vi "CRYAnalysis.vi"(0 "Setup in":T3={"No.VI"=0, "Category"="", "StepName"="", "Seq setup flattened"="", "Comment"="", "Steps config."=[], "Jump config"=[], "Start"=0.0, "Increment"=0.0, "Name"="Pa", "Unit"="Pa", "Y data"=1, "Y prefix"="", "Y dB ref"=1.0, "Y unit"="", "Repeat State Array"=[]} {"Repeat State Array"."Start" format="%#_5g"; "Y dB ref" format="%.1f"; "Y data" items=["dB", "Lin"]; "Start" format="%#_5g"}, 5 "Data in":T8 {"Z data" items=["dB", "Lin"]; "X data" items=["dB", "Lin"]; "Y data" items=["dB", "Lin"]; "Z dB ref" format="%.1f"; "Z axis" items=["Log", "Lin"]; "X dB ref" format="%.1f"; "X axis" items=["Log", "Lin"]; "Y axis" items=["Log", "Lin"]; "Y dB ref" format="%.1f"; "Curve"."z" format="%.2f"; "Curve"."y" format="%.2f"; "Curve"."x" format="%.2f"}, 7 "Results in":T9 {"Margin" format="%.2f"}, 9 "Seq Setup in":string, 11 "Step name":string, 12 "Hardware in":string, 13 "Calibration in":string) -> (3 "Types Out":string[](array[string]), 4 "Inserted Names Out":string[](array[string]), 6 "Data out":T8 {"Z data" items=["dB", "Lin"]; "X data" items=["dB", "Lin"]; "Y data" items=["dB", "Lin"]; "Z dB ref" format="%.1f"; "Z axis" items=["Log", "Lin"]; "X dB ref" format="%.1f"; "X axis" items=["Log", "Lin"]; "Y axis" items=["Log", "Lin"]; "Y dB ref" format="%.1f"; "Curve"."z" format="%.2f"; "Curve"."y" format="%.2f"; "Curve"."x" format="%.2f"}, 8 "Results out":T1[](array[typedef]) {"Margin" format="%.2f"}, 10 "Wave out":T7[](array[typedef]) {"Y dB ref" format="%.1f"; "Y axis" items=["Log", "Lin"]; "Y data" items=["dB", "Lin"]; "X data" items=["dB", "Lin"]})   [LabVIEW 2013]
doc: "This VI calculates the Vrms response of a device under test to a series of stepped inputs. It is designed to be used with the create stepped sign waveform.vi. The output is a 2-D array of Vrms data. Rows refer to the channel sampled. Columns refer to each step in the test signal. The user can elect to discard some number of cycles at the beginning of each frequency."
uses:
  Typedef Control/CRYData Cluster Array.ctl
  Typedef Control/CRYData Cluster.ctl
  Typedef Control/CRYResult Cluster Array.ctl
  Typedef Control/CRYResult Cluster.ctl
  Typedef Control/CRYWaveform Cluster.ctl
  Typedef Control/CRYUnit Info Cluster.ctl
  Typedef Control/CRYCalibration 2DCluster.ctl
  Typedef Control/CRYCalibration Cluster.ctl
  Typedef Control/CRYStep.ctl
  Typedef Control/CRYStimulus Test Infor Cluster.ctl
  CRYMainGlobal.vi
  Task Sequence/CRYProject Run Control Global.vi
  Calibration/SubVI/CRYCal Global.vi
  Hardware/SubVI/CRY6175APT_Win32.dll
panel:
  out "XY Graph":cluster{dbl[], dbl[]}(graph)
  in  "Result":T1={"Name"="Test for Signal [L]", "Margin"=nan, "unit"="", "Verdict"=FALSE, "Limit"="", "Max/Min"="", "protected"=FALSE, "Step No."=0, "Test Info"="", "AutoProtect"=FALSE} {"Margin" format="%.2f"}
  in  "Datum":T2={"Name"="", "Curve"=[], "X data"=1, "Y data"=1, "Z data"=1, "X axis"=0, "Y axis"=1, "Z axis"=1, "X unit"="", "Y unit"="", "Z unit"="", "X dB ref"=1.0, "Y dB ref"=1.0, "Z dB ref"=1.0, "single val"=FALSE, "protected"=FALSE, "display X"=TRUE, "display Y"=FALSE, "display Z"=TRUE, "Test Info"="", "Step No."=0, "Plot Settings"={"Color"=0, "Interpolation"=0, "Point Style"=0, "Line Style"=0, "Point Color"=0, "Line Width"=0, "Bar Plot Style"=0, "Fill To"=0}, "AutoProtect"=FALSE} {"Z data" items=["dB", "Lin"]; "X data" items=["dB", "Lin"]; "Y data" items=["dB", "Lin"]; "Z dB ref" format="%.1f"; "Z axis" items=["Log", "Lin"]; "X dB ref" format="%.1f"; "X axis" items=["Log", "Lin"]; "Y axis" items=["Log", "Lin"]; "Y dB ref" format="%.1f"; "Curve"."z" format="%.2f"; "Curve"."y" format="%.2f"; "Curve"."x" format="%.2f"}
  out "Response Waveform":waveform(dbl)(graph)
  in  "Calibration All Cluster":T4={"Calibration"={"Calibration Step Name"="", "Device"="", "Correction Curve Name"="", "Equalization Curve Name"="", "Sensitivity Curve Name"="", "Corr Folder and File"="", "EQ Folder and File"="", "Sens Folder and File"="", "Corr Step size"=0, "EQ Step size"=0, "Input"=FALSE, "Last Cal Date (sec)"=timestamp(0 s since 1904-01-01), "Cha Name"="", "Corr Curve Found"=FALSE, "EQ Curve Found"=FALSE, "Sens Curve Found"=FALSE, "Signal Type"="", "Calibrated Device"="", "Hz"=0}, "Corr Curve"={"Name"="", "Curve"=[], "X data"=1, "Y data"=1, "Z data"=1, "X axis"=0, "Y axis"=1, "Z axis"=1, "X unit"="", "Y unit"="", "Z unit"="deg.", "X dB ref"=1.0, "Y dB ref"=1.0, "Z dB ref"=1.0, "single val"=FALSE, "protected"=FALSE, "display X"=FALSE, "display Y"=TRUE, "display Z"=TRUE, "Test Info"="", "Step No."=0, "Plot Settings"={"Color"=0, "Interpolation"=0, "Point Style"=0, "Line Style"=0, "Point Color"=0, "Line Width"=0, "Bar Plot Style"=0, "Fill To"=0}, "AutoProtect"=FALSE}, "EQ Curve"={"Name"="", "Curve"=[], "X data"=1, "Y data"=1, "Z data"=1, "X axis"=0, "Y axis"=1, "Z axis"=1, "X unit"="Hz", "Y unit"="", "Z unit"="deg.", "X dB ref"=1.0, "Y dB ref"=1.0, "Z dB ref"=1.0, "single val"=FALSE, "protected"=FALSE, "display X"=TRUE, "display Y"=TRUE, "display Z"=TRUE, "Test Info"="", "Step No."=0, "Plot Settings"={"Color"=0, "Interpolation"=0, "Point Style"=0, "Line Style"=0, "Point Color"=0, "Line Width"=0, "Bar Plot Style"=0, "Fill To"=0}, "AutoProtect"=FALSE}, "Sens Curve"={"Name"="", "Curve"=[], "X data"=1, "Y data"=1, "Z data"=1, "X axis"=0, "Y axis"=1, "Z axis"=1, "X unit"="Hz", "Y unit"="", "Z unit"="deg.", "X dB ref"=1.0, "Y dB ref"=1.0, "Z dB ref"=1.0, "single val"=FALSE, "protected"=FALSE, "display X"=TRUE, "display Y"=TRUE, "display Z"=TRUE, "Test Info"="", "Step No."=0, "Plot Settings"={"Color"=0, "Interpolation"=0, "Point Style"=0, "Line Style"=0, "Point Color"=0, "Line Width"=0, "Bar Plot Style"=0, "Fill To"=0}, "AutoProtect"=FALSE}} {"Sens Curve"."Z data" items=["dB", "Lin"]; "Sens Curve"."X data" items=["dB", "Lin"]; "Sens Curve"."Y data" items=["dB", "Lin"]; "Sens Curve"."Z dB ref" format="%.1f"; "Sens Curve"."Z axis" items=["Log", "Lin"]; "Sens Curve"."X dB ref" format="%.1f"; "Sens Curve"."X axis" items=["Log", "Lin"]; "Sens Curve"."Y axis" items=["Log", "Lin"]; "Sens Curve"."Y dB ref" format="%.1f"; "Sens Curve"."Curve"."z" format="%.2f"; "Sens Curve"."Curve"."y" format="%.2f"; "Sens Curve"."Curve"."x" format="%.2f"; "EQ Curve"."Z data" items=["dB", "Lin"]; "EQ Curve"."X data" items=["dB", "Lin"]; "EQ Curve"."Y data" items=["dB", "Lin"]; "EQ Curve"."Z dB ref" format="%.1f"; "EQ Curve"."Z axis" items=["Log", "Lin"]; "EQ Curve"."X dB ref" format="%.1f"; "EQ Curve"."X axis" items=["Log", "Lin"]; "EQ Curve"."Y axis" items=["Log", "Lin"]; "EQ Curve"."Y dB ref" format="%.1f"; "EQ Curve"."Curve"."z" format="%.2f"; "EQ Curve"."Curve"."y" format="%.2f"; "EQ Curve"."Curve"."x" format="%.2f"; "Corr Curve"."Z data" items=["dB", "Lin"]; "Corr Curve"."X data" items=["dB", "Lin"]; "Corr Curve"."Y data" items=["dB", "Lin"]; "Corr Curve"."Z dB ref" format="%.1f"; "Corr Curve"."Z axis" items=["Log", "Lin"]; "Corr Curve"."X dB ref" format="%.1f"; "Corr Curve"."X axis" items=["Log", "Lin"]; "Corr Curve"."Y axis" items=["Log", "Lin"]; "Corr Curve"."Y dB ref" format="%.1f"; "Corr Curve"."Curve"."z" format="%.2f"; "Corr Curve"."Curve"."y" format="%.2f"; "Corr Curve"."Curve"."x" format="%.2f"; "Calibration"."EQ Step size" items=["R10", "R20", "R40", "R80", "User"]; "Calibration"."Corr Step size" items=["R10", "R20", "R40", "R80", "User"]}
  out "Impulse Resp Y":dbl[][](array[numeric]) format="%.2f"
  out "Impulse Resp X":dbl[](array[numeric]) format="%.2f"
  out "Unit Info":T6
  out "Y dB ref Curve":dbl
  out "Y dB ref In":dbl
  out "Y dB ref Out":dbl
  out "Y unit Out":string
  out "Y unit In":string
  out "Sens Out":dbl format="%.2f"
  out "Freq Option":bool[](array[boolean])
  out "Channel Label In":string
  out "TSR window":u16
  in  "AC/DC":i32(slide)
  out "Stimulus Waveform":waveform(dbl)(graph)
  out "HT Option":bool[](array[boolean])
  out "Window":u16
  out "Spectrum X-axis":dbl[](array[numeric]) format="%.2f"
  in  "Manual?":bool
  in  "Y data Curve":u16(ring)=1 items=["dB", "Lin"]
  out "Y Unit Curve":string
  in  "Ref resistor":dbl format="%.2f"
  out "Sens In":dbl format="%.2f"
  out "Analysis Settings":bool
  out "Input":bool
  in  "Frequency [Hz]":dbl[](array[numeric]) format="%.2f"
  in  "cycles":u32=12
  in  "Response Data":dbl[](array[numeric]) format="%.2e"
  # "V"
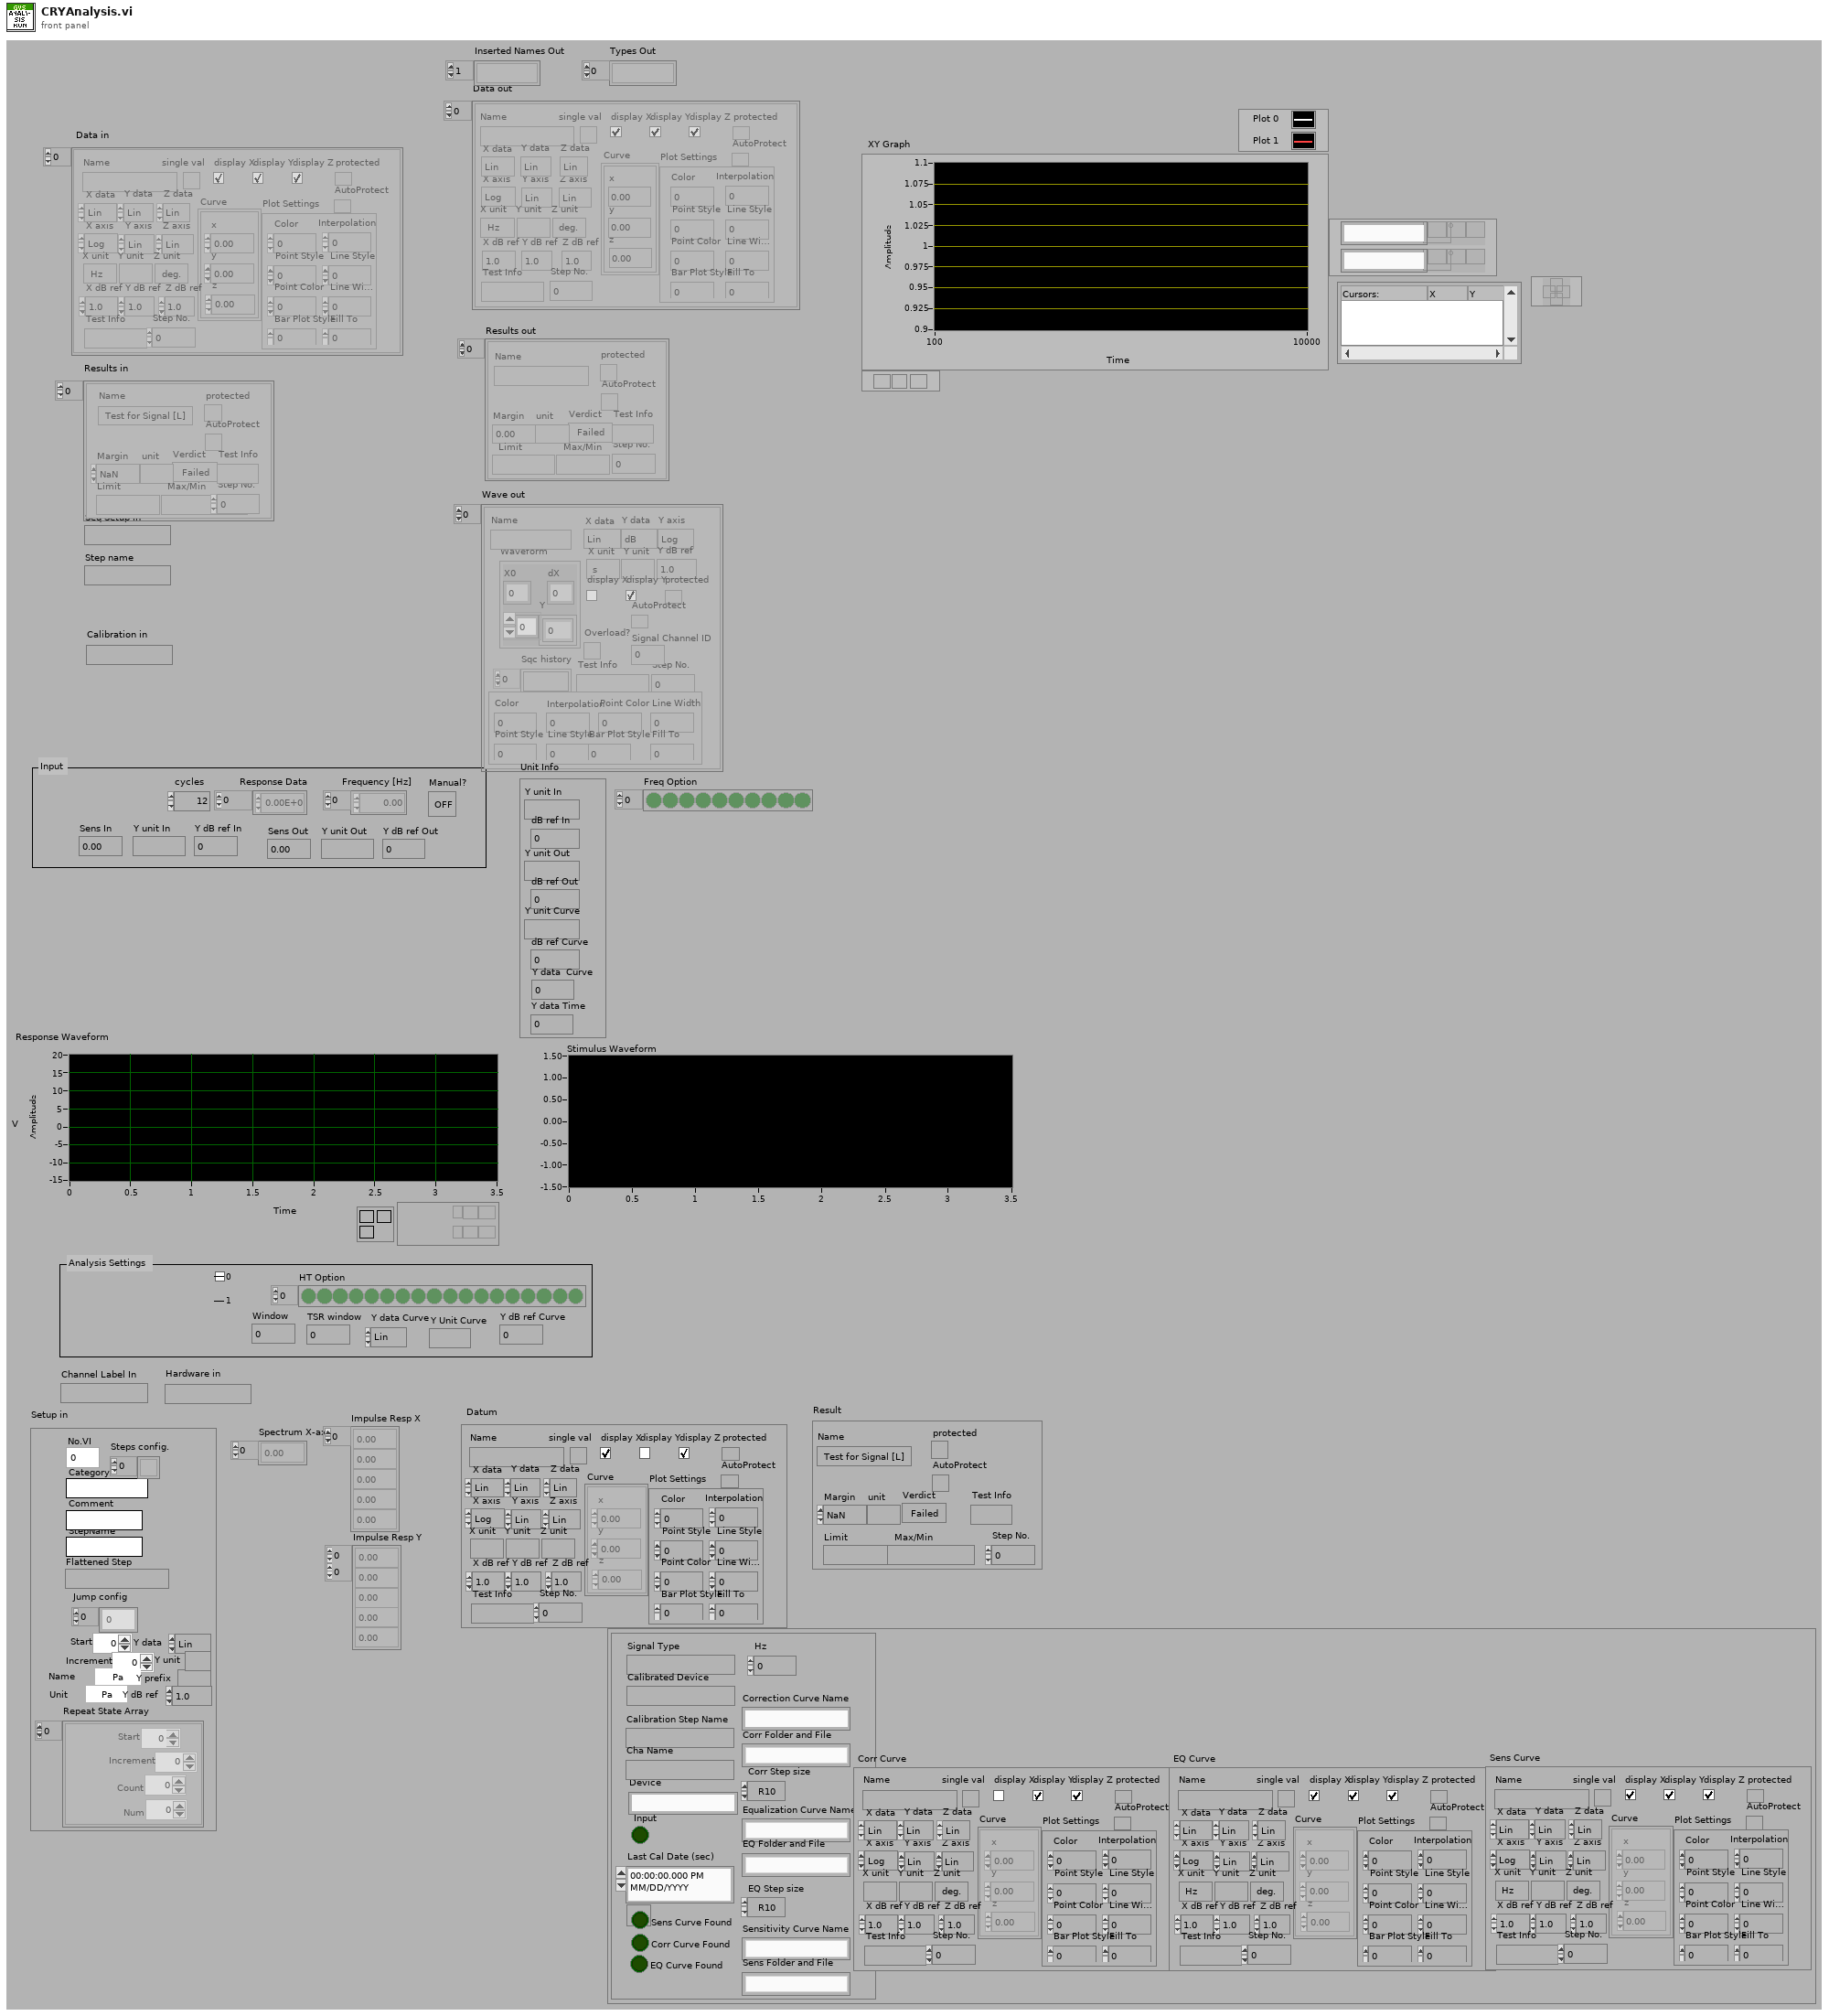
[diagram p1: front panel]
types:
  T1 = typedef "CRYResult Cluster.ctl" = cluster{"Name":string, "Margin":dbl, "unit":string, "Verdict":bool, "Limit":string, "Max/Min":string, "protected":bool, "Step No.":i32, "Test Info":string, "AutoProtect":bool}
  T2 = typedef "CRYData Cluster.ctl" = cluster{"Name":string, "Curve":cluster{"x":dbl, "y":dbl, "z":dbl}[], "X data":u16, "Y data":u16, "Z data":u16, "X axis":u16, "Y axis":u16, "Z axis":u16, "X unit":string, "Y unit":string, "Z unit":string, "X dB ref":dbl, "Y dB ref":dbl, "Z dB ref":dbl, "single val":bool, "protected":bool, "display X":bool, "display Y":bool, "display Z":bool, "Test Info":string, "Step No.":i32, "Plot Settings":cluster{"Color":u32, "Interpolation":u8, "Point Style":u8, "Line Style":u8, "Point Color":u32, "Line Width":u8, "Bar Plot Style":u8, "Fill To":i16}, "AutoProtect":bool}
  T3 = typedef "CRYStep.ctl" = cluster{"No.VI":i32, "Category":string, "StepName":string, "Seq setup flattened":string, "Comment":string, "Steps config.":bool[], "Jump config":i32[], "Start":dbl, "Increment":dbl, "Name":string, "Unit":string, "Y data":u16, "Y prefix":string, "Y dB ref":dbl, "Y unit":string, "Repeat State Array":cluster{"Start":dbl, "Increment":dbl, "Count":i32, "Num":i32}[]}
  T4 = typedef "CRYCalibration 2DCluster.ctl" = cluster{"Calibration":T5, "Corr Curve":T2, "EQ Curve":T2, "Sens Curve":T2}
  T5 = typedef "CRYCalibration Cluster.ctl" = cluster{"Calibration Step Name":string, "Device":string, "Correction Curve Name":string, "Equalization Curve Name":string, "Sensitivity Curve Name":string, "Corr Folder and File":string, "EQ Folder and File":string, "Sens Folder and File":string, "Corr Step size":u16, "EQ Step size":u16, "Input":bool, "Last Cal Date (sec)":timestamp, "Cha Name":string, "Corr Curve Found":bool, "EQ Curve Found":bool, "Sens Curve Found":bool, "Signal Type":string, "Calibrated Device":string, "Hz":u32}
  T6 = typedef "CRYUnit Info Cluster.ctl" = cluster{"Y unit In":string, "dB ref In":dbl, "Y unit Out":string, "dB ref Out":dbl, "Y unit Curve":string, "dB ref Curve":dbl, "Y data  Curve":u16, "Y data Time":u16}
  T7 = typedef "CRYWaveform Cluster.ctl" = cluster{"Waveform":cluster{"X0":dbl, "dX":dbl, "Y":sgl[]}, "X data":u16, "Y data":u16, "Y axis":u16, "X unit":string, "Y unit":string, "Y dB ref":dbl, "display Y":bool, "display X":bool, "Overload?":bool, "Test Info":string, "Step No.":i32, "Name":string, "protected":bool, "Sqc history":string[], "Signal Channel ID":i32, "Plot Settings":cluster{"Color":u32, "Interpolation":u8, "Point Style":u8, "Line Style":u8, "Point Color":u32, "Line Width":u8, "Bar Plot Style":u8, "Fill To":i16}, "AutoProtect":bool}
  T8 = typedef "CRYData Cluster Array.ctl" = T2[]
  T9 = typedef "CRYResult Cluster Array.ctl" = T1[]
  T10 = cluster{"Start":dbl, "Increment":dbl, "Count":i32, "Num":i32}[]
  T11 = enum16{"OK", "Yes", "YesNo", "YesNoCancel", "ReplaceAppend"}
  T12 = cluster{"Harmonic Track Data":cluster{cluster{"x":dbl, "y":dbl, "z":dbl}[]}[]}[]
  T13 = typedef "CRYAnalysis Cluster.ctl" = cluster{"Name":string, "Harmonics":dbl[], " Algorithm":u16, "delay":dbl, "THD(%)":bool, "Rub&Buzz":bool, "Imp":bool, "Imp Ref resistor":dbl, "Y data":u16, "Y prefix":string, "Y unit":string, "Y dB ref":dbl, "Custom Curve Names":string[], "har list items":string[], "Envelope":bool, "use custom unit":bool, "autodelay ch":dbl, "impulse":bool, " start ms":dbl, " stop ms":dbl, "Scaling":i32, "Default Overlap ":bool, "Advanced View":bool, "Loose Particle":bool, "Use default":bool, "Auto-Correlation(Stimulus)":bool, "Auto-Correlation(Response)":bool, "Deconvolved Response":bool, "Mic Current":bool, "M List Vaiues":u16, "Type":u16, "Delay Method":u16, "Apply Correction Out":bool, "Apply Correction In":bool, "Harmonics @ meas.frq":bool, "THD Normalized(%)":bool, "Total Distortion":bool, "THD+Noise(%)":bool, "Rub&Buzz Norm'd(%)":bool, "Standard Error":bool, "Confidence Limits":bool, "Total Diff":bool, "Total Noise":bool, "Total DFD(%)":bool, "Total IMD(%)":bool, "Total IM":bool, "Total DFD+Noise(%)":bool, "Use Channel Name":bool, "Waveform In":string, "Waveform Out":string, "Method":u16, "Spectral Scaling":u16, "Appliied Unit":u16, "Length Unit":u16, "Applied Units":u16, "Sens Item":u16, "Tab":i32, "Distance Unit":u16, "discard cycles":dbl, "Weigting":string, "Averaging Time":dbl, "Max duration":dbl, "Min duration":dbl, "Attack Threshold":dbl, "Hysteresis Up":dbl, "Fmin(Hz)":dbl, "Fmax(Hz)":dbl, "Freq.Resolution":dbl, "Over-samples Res.":dbl, "Win Resolution":dbl, "distance":dbl, "samples":dbl, "Overlap":dbl, "Record Length":dbl, "No.of FFTs":dbl, "Hz":dbl, "record delay":dbl, " Std Err":dbl, "Response":bool, "Coherent Power*":bool, "Stimulus":bool, "Measurement Confidence":bool, "Auto Spectrum(Response)*":bool, "Auto Spectrum(Stimulus)*":bool, "Cross Spectrum*":bool, "functions":bool, "Frequency Response":bool, "Non-Coherent Power*":bool, "Coherence (%)":bool, "Non-Coherence (%)":bool, "Signal-Noise Ratio (dB)":bool, "Non-Coherenct Distirtion*":bool, "Result Waveforms":bool, "Coupling":bool, "Averaging":u16, "Harmonics":i32, "Custom Curve Names":i32, "unLabel":string, "Custom Curve Names":string, "Unit":string, "Total IMD + Noise(%) ":bool, "ResponseMe":u16, "Intermod":dbl[], "Diff\n":dbl[], "Cross-Correlation":bool, "IM list items":string[], "Diff list items":string[], "TSR Window Type":string, "Help":string, "Custom Curve IDs":i32[], "Default Curve Names":string[], "Loose Particle waveform":bool, "Perceptual Rub&Buzz":bool, "Imp Auto Mode":u16, "Mic Auto Mode":u16, "Mic Ref resistor":dbl, "Curve Resolution":u16, "Curve Resolution Hz":dbl, "Polarity":bool}
  T14 = typedef "CRYStimulus Test Infor Cluster.ctl" = cluster{"Stimulus Type":string, "Signal Type":string, "In/Out":bool, "FAPS":cluster{"freq":dbl, "ampl":dbl, "cycles":dbl, "samples":i32}[], "Sampling Rate":dbl, "Samples":i32, "Analysis Param":string, "Resolution":u16, "Steps":u32, "Analysis Value":dbl[], "Diff Freq":dbl, "FStart":dbl, "FStop":dbl, "Calibration Param":string, "Anti Alias":dbl, "Level Out1":dbl, "Level Out2":dbl, "EQ":bool}
  T15 = cluster{bool, "Check Option":string, "use custom unit":bool, "Custom Curve Names":string[], "Custom Curve IDs":i32[], "Default Curve Names":string[], "Use default":bool}
  T16 = cluster{"freq":dbl, "ampl":dbl, "cycles":dbl, "samples":i32}[]
  T17 = cluster{"Y unit":string, "Y dB ref":dbl, "Y unit":string, "Y dB ref":dbl, "Y unit":string, "Y dB ref":dbl, "Y data":u16, u16}
  T18 = cluster{"Sampling Rate":dbl, "discard cycles":dbl, "Sens In":dbl, "AC/DC":i32}
  T19 = cluster{"Window":u16, "Freq.Resolution":dbl, "Overlap":dbl, "Spectral Scaling":u16, "Sens In":dbl}
  T20 = cluster{"EQ Curve":T2, "EQ":bool, "Level Out2":dbl}
  T21 = cluster{"ResponseMe":u16, "Sampling Rate":dbl, "Sens In":dbl}
  T22 = cluster{dbl[], "Frequency [Hz]":dbl[], dbl[], bool, "Diff Freq":dbl}
  T23 = cluster{"Type":u16, "Method":u16, "HT Option":bool[], "Harmonics array out":dbl[], bool, "Apply Correction In":bool, " Std Err":dbl}
  T24 = cluster{dbl[], "Frequency [Hz]":dbl[], dbl[], i32[], "Sampling Rate":dbl, "Window":u16, "discard cycles":dbl}
  T25 = cluster{"FSamp":dbl, "FStart":dbl, "FStop":dbl, "NOffset":dbl, "MStop":dbl, "MStart":dbl, "NHarm":dbl, "Tsamp":dbl, "Amplit":dbl, "Amplit 2":dbl}
  T26 = cluster{"TSR Window Type":string, " start ms":dbl, " stop ms":dbl, "Over-samples Res.":dbl}
  T27 = cluster{dbl[], dbl[], dbl[], i32[], "Sampling Rate":dbl, "Window":u16, "Sampling Rate":dbl}
  T28 = cluster{"Curve Resolution Hz":dbl, "Overlap":dbl, "Window":u16}
  T29 = cluster{"display X":bool, "display Y":bool, "display Z":bool}[]
  T30 = typedef "CRYUnit Info Out Cluster.ctl" = cluster{"X unit":string, "X data":u16, "Y unit":string, "Y data Time":u16, "Z unit":string, "X axis":u16, "X dB ref":dbl, "Y dB ref":dbl, "single/curve":bool}
  T31 = typedef "CRYAnalysis CurveName Cluster.ctl" = cluster{"Custom Curve Name":string, "Custom Curve ID":i32, "Default Curve Name":string}[]
  T32 = cluster{bool, "Check Option":string, bool, "Custom Curve Names":string[], "Custom Curve IDs":i32[], "Default Curve Names":string[], "Use default":bool}
  T33 = cluster{"display X":bool, "display Y":bool, "display Z":bool}
  T34 = cluster{"Harmonics array out":dbl[], "Impulse Resp X":dbl[], "Impulse Resp Y":dbl[][]}
  T35 = cluster{"Fmin(Hz)":dbl, "Fmax(Hz)":dbl, "Averaging":u16, "Scaling":i32}
  T36 = cluster{"Sampling Rate":dbl, "Channel Label In":string, "Make Fundamental curve?":bool}
  T37 = cluster{"Window":u16, "TSR window":u16, "Freq.Resolution":dbl, "Default Overlap ":bool, "Overlap":dbl, "discard cycles":dbl, " start ms":dbl, " stop ms":dbl, "Over-samples Res.":dbl, "ResponseMe":u16, "Weigting":string}
  T38 = cluster{bool, string, "use custom unit":bool, "Custom Curve Names":string[], "Custom Curve IDs":i32[], "Default Curve Names":string[], "Use default":bool}
  T39 = cluster{"Attack Threshold":dbl, "Averaging Time":dbl, "Max duration":dbl, "Min duration":dbl, "Hysteresis Up":dbl, "Loose Particle":bool}
  T40 = typedef "CRYWaveform Cluster Array.ctl" = T7[]
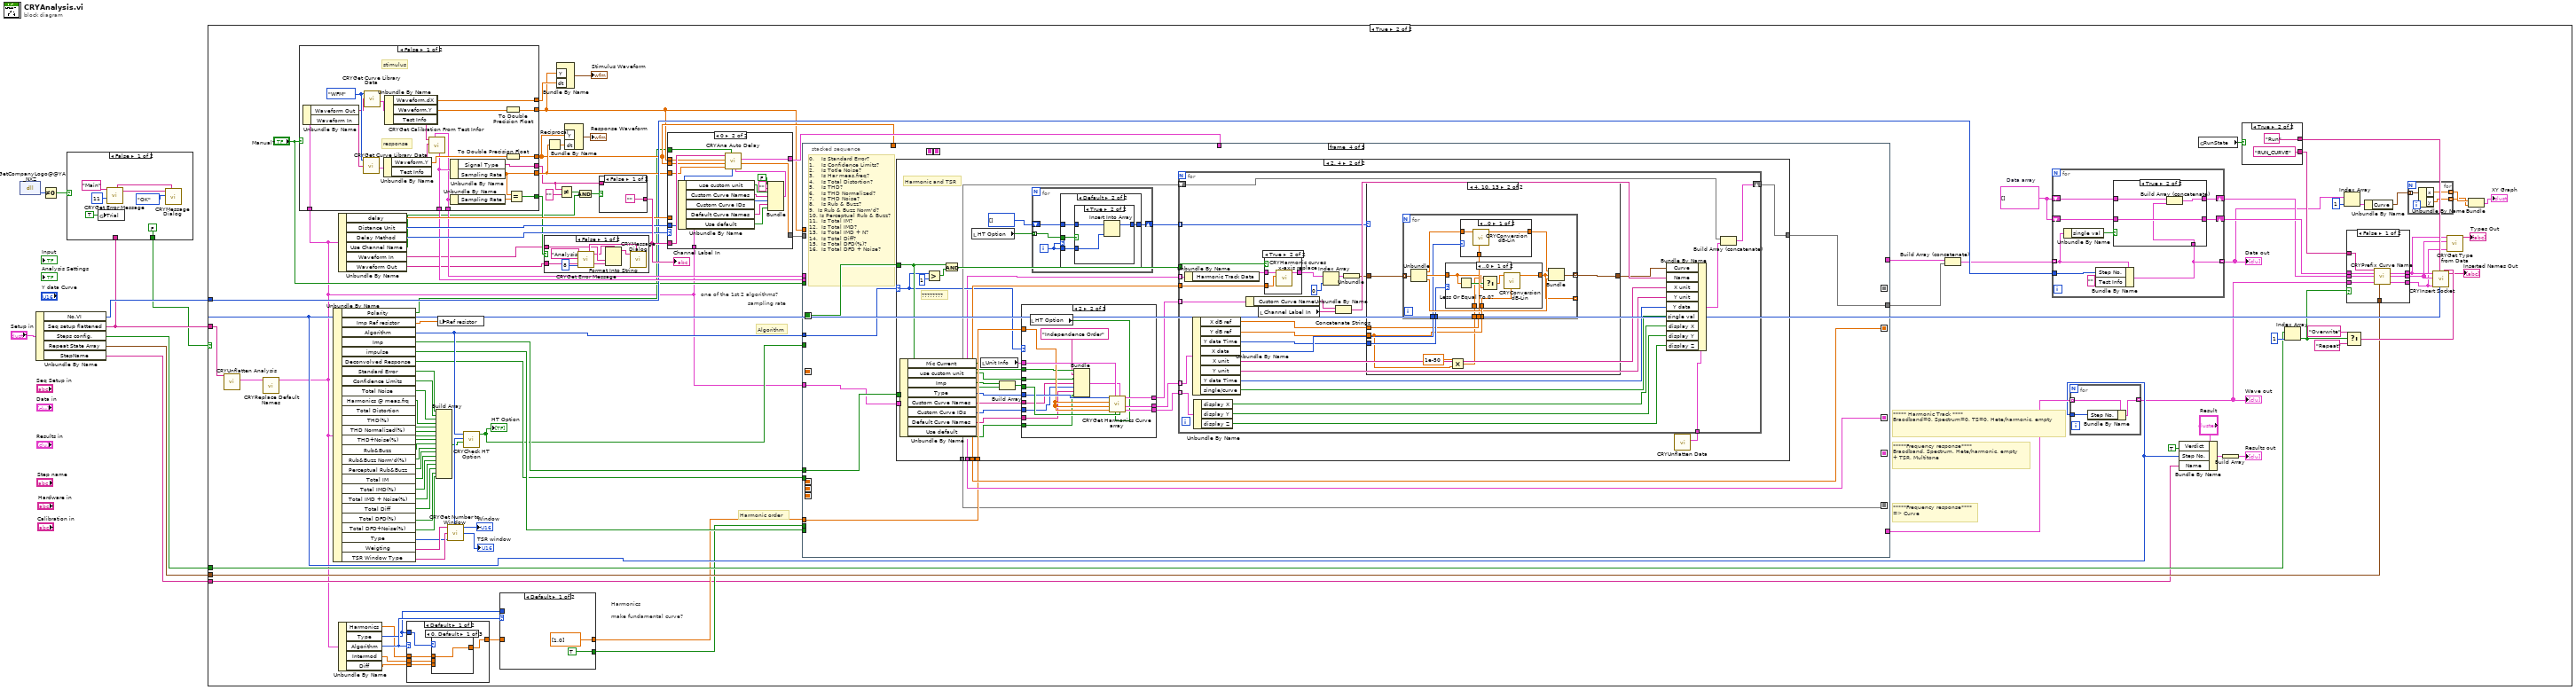
[diagram p0: block diagram]
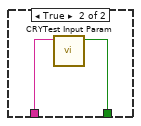
[diagram p2: hidden frame]
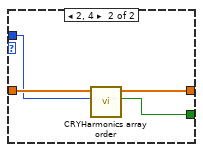
[diagram p4: hidden frame]
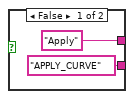
[diagram p6: hidden frame]
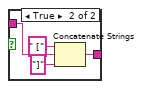
[diagram p8: hidden frame]
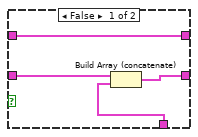
[diagram p9: hidden frame]
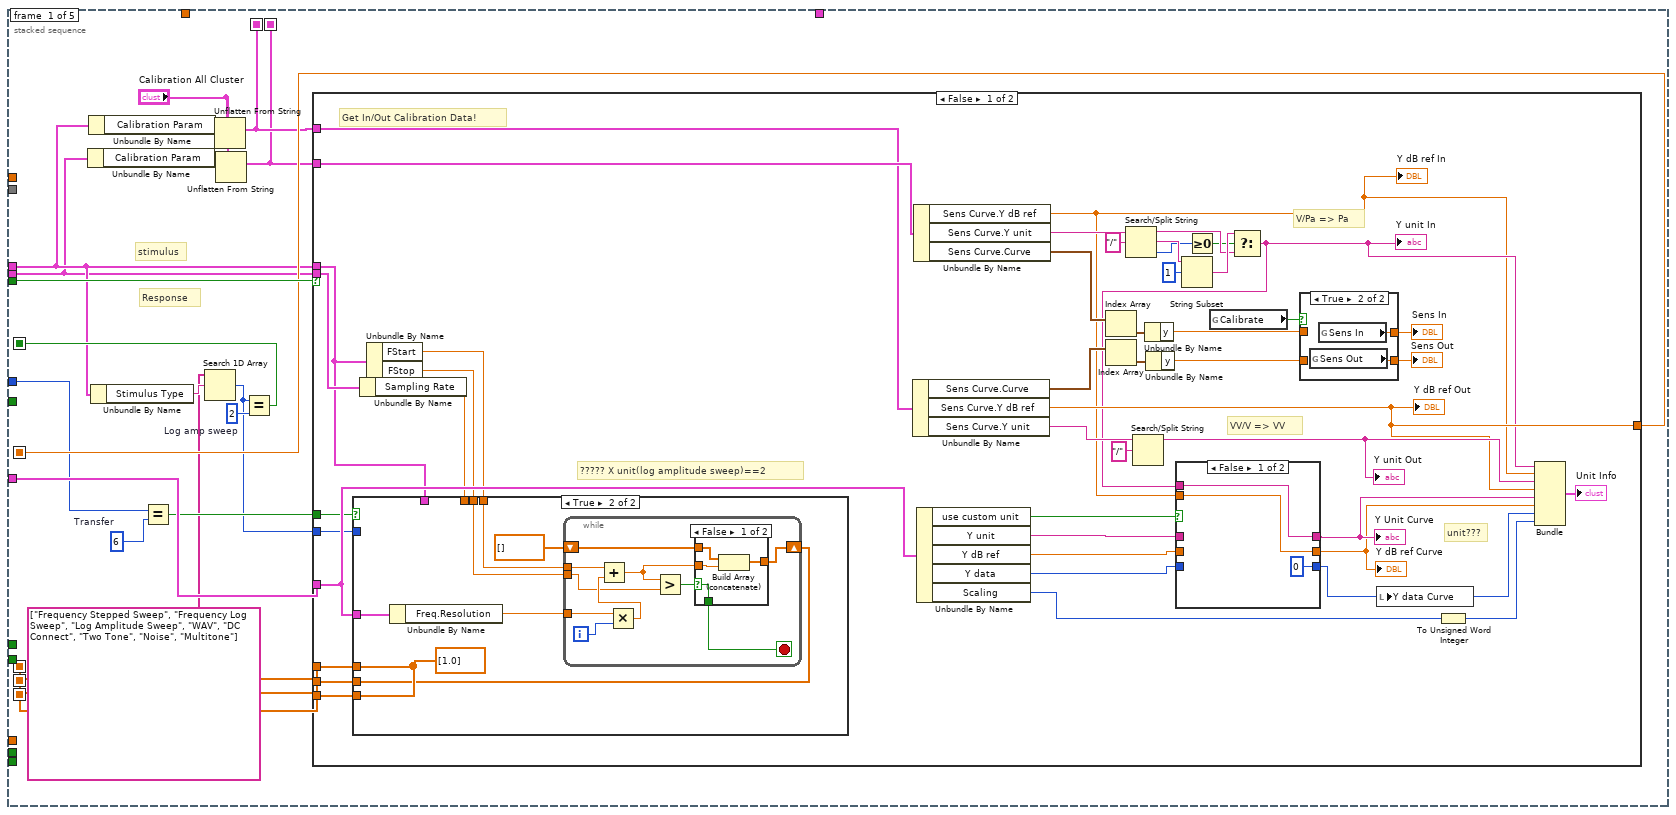
[diagram p10: hidden frame]
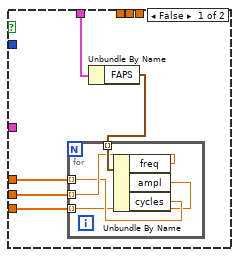
[diagram p11: hidden frame]
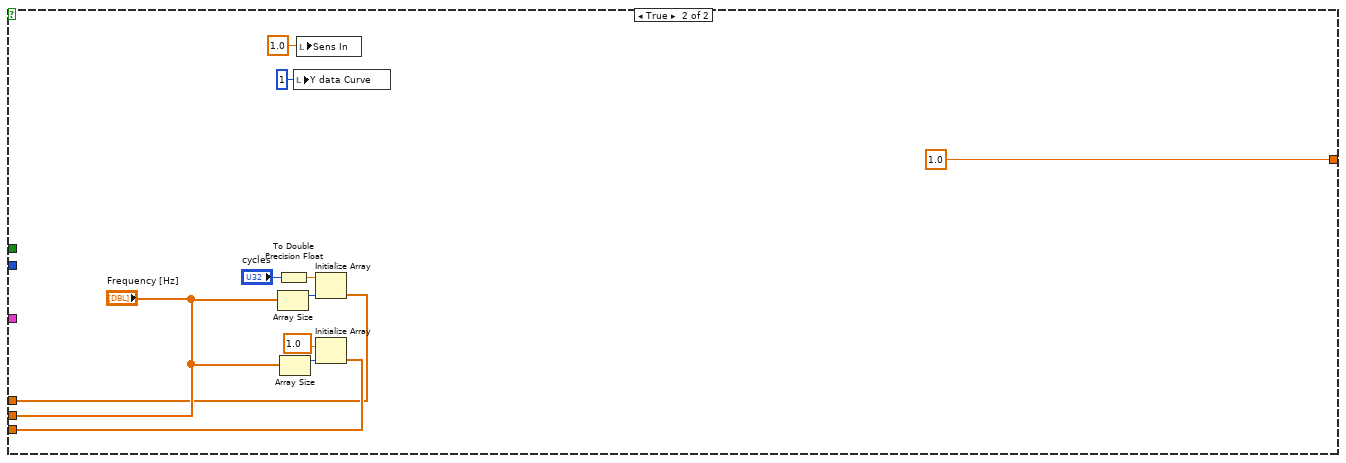
[diagram p15: hidden frame]
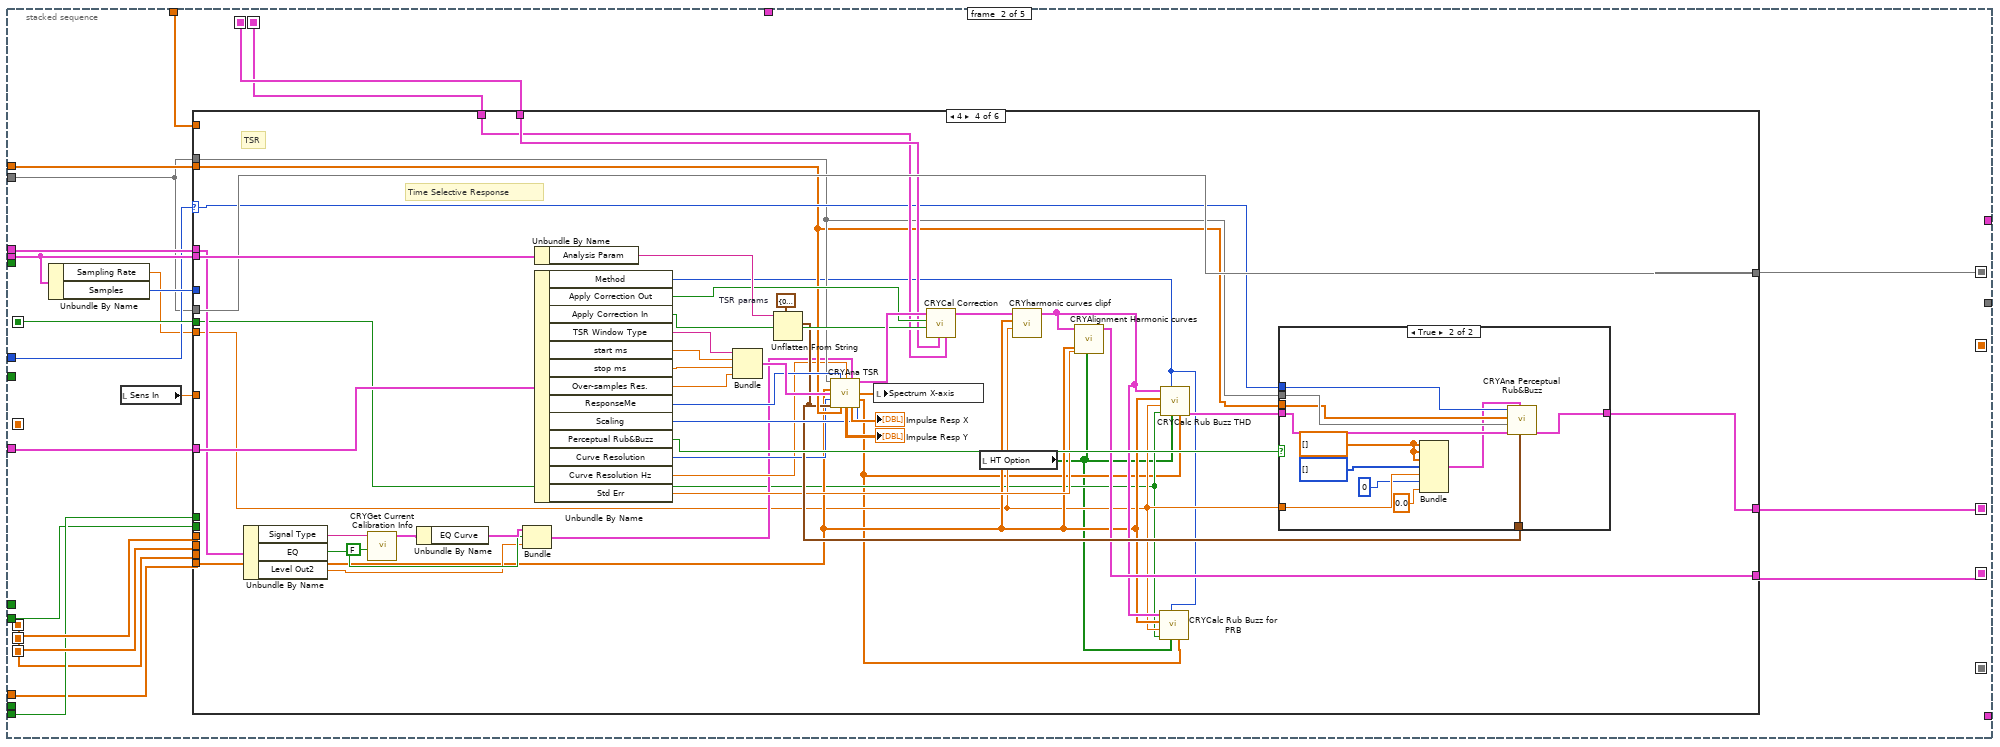
[diagram p16: hidden frame]
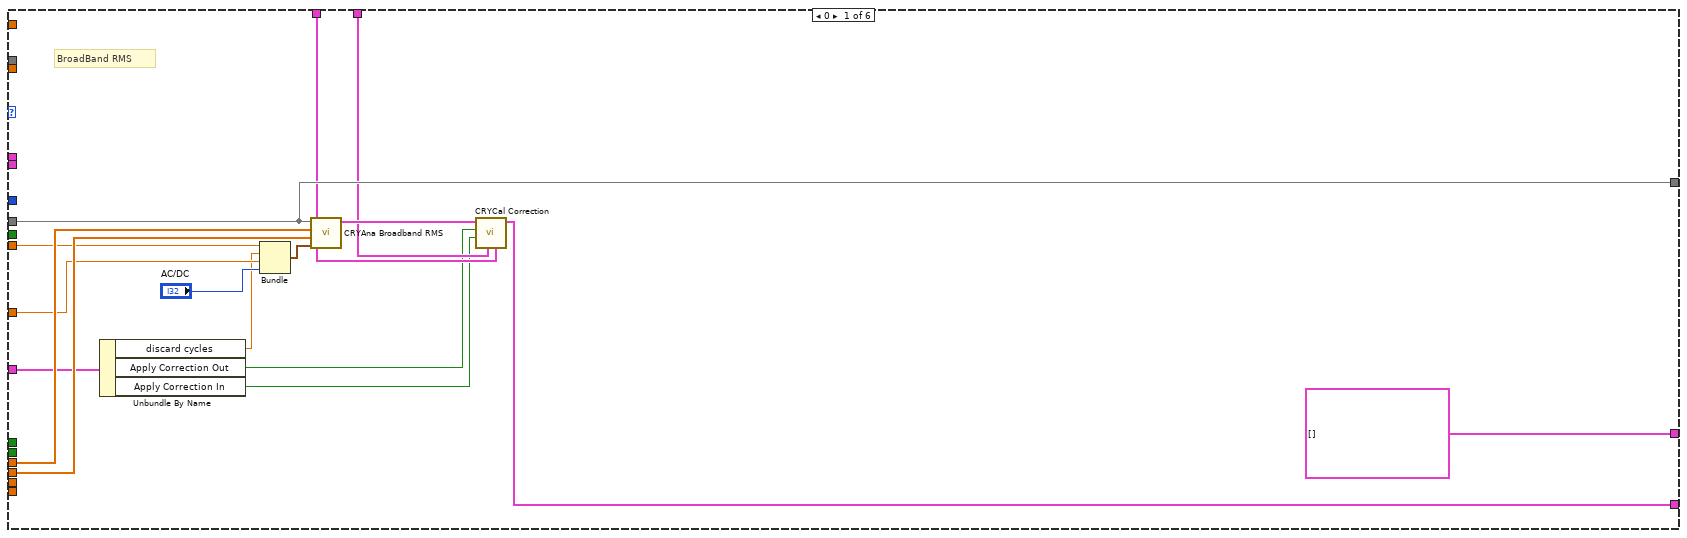
[diagram p17: hidden frame]
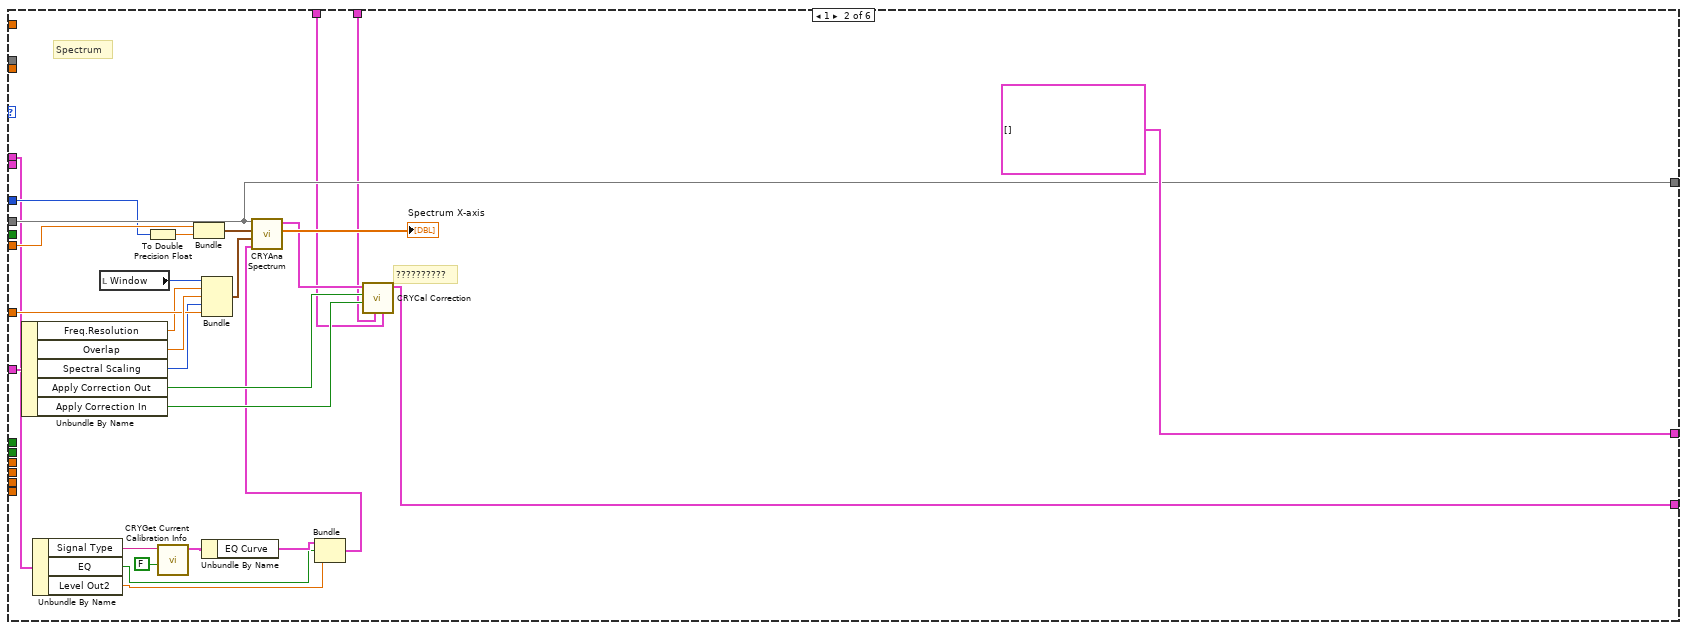
[diagram p18: hidden frame]
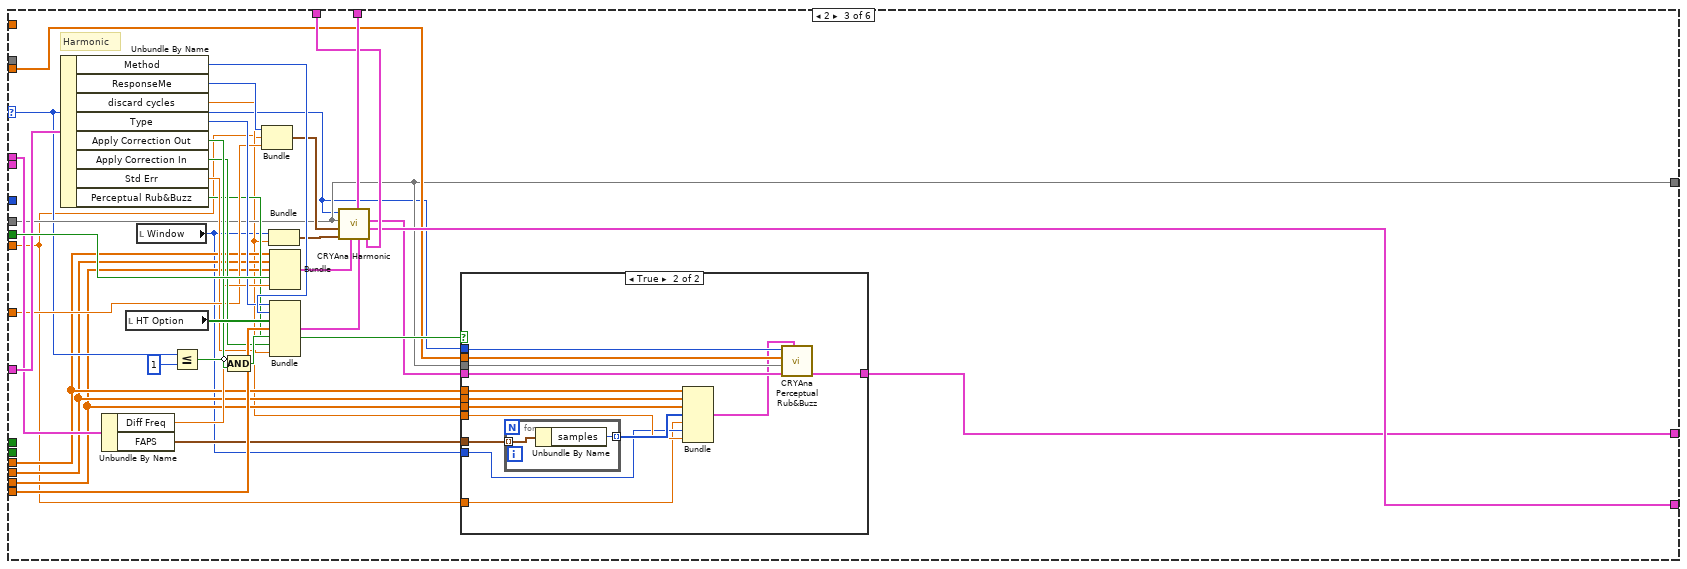
[diagram p19: hidden frame]
diagram:
  n1 = dll-call lib="D:/A_CRYSoundLab_Work/CRY6181/CRYSystem/Hardware/SubVI/CRY6175APT_Win32.dll" fn="?GetCompanyLogo@@YA_NXZ"() -> ("return type"=w4:i32)  [unwired: 3 in, 2 out]
  n2 = Unbundle By Name("Setup in") -> ("No.VI"=w9:i32, "Seq setup flattened"=w2:string, "Steps config."=w8:bool[], "Repeat State Array"=w7:T10, "StepName"=w6:string)
  n3 = Not Equal To 0?(x=w4) -> (x != 0?=w3:bool)
  n4 = case shown="False" w3 {
    tunnel: w2 -> [_ w18]
    tunnel: [FALSE ("test result") w17] -> w1
    frame False {
      n5 = global write "CRYMainGlobal.vi" "Trial"(TRUE ("Trial")) -> ()
      n6 = call "CRYGet Error Message.vi"("Error No"=11, "Kind"="Main") -> ("Message"=w11:string, "Window Title"=w15:string)  [unwired: 4 in, 4 out]
      n7 = call "CRYMessage Dialog.vi"("Window Title"=w15, "YesNoCancel"=T11."OK", "Message Content"=w11) -> ()  [unwired: 7 in, 2 out]
    }
    frame True {
      n8 = call "CRYTest Input Param.vi"("Flattend Analysis"=w18) -> ("test result"=w17:bool)  [unwired: 10 out]
    }
  }
  n9 = case shown="True" w1 {
    tunnel: w9 -> [_ w101]
    tunnel: w8 -> [_ w97]
    tunnel: w7 -> [_ w90]
    tunnel: w6 -> [_ w45]
    tunnel: w2 -> [_ w27]
    frame False {
    }
    frame True {
      w48 = T8 []  # Data array
      # "make fundamental curve?"
      # "Harmonics"
      # "*****Frequency response****\n=> Curve"
      # "***** Harmonic Track ****\nBraodband=0, Spectrum=0, TS=0, Hete/harmonic, empty"
      # "*****Frequency response****\nBraodband, Spectrum, Hete/harmonic, empty\n+ TSR, Multitone"
      # "Harmonic order"
      # "sampling rate"
      # "Algorithm"
      # "one of the 1st 2 algorithms?"
      n10 = call "CRYUnflatten Analysis.vi"("Unflatten Analysis"=w27) -> ("Analysis"=w25:T13)  [unwired: 10 out]
      n11 = call "CRYReplace Default Names.vi"("Analysis In"=w25) -> ("Analysis Out"=w24:T13)  [unwired: 10 in]
      n12 = case shown="False" "Manual?" {
        tunnel: [w1181 "Response Data"] -> w29
        tunnel: [w1182 "Response Data"] -> w94
        tunnel: w24 -> [w1180 _]
        tunnel: [w1179 "" ("Stimulus Type")] -> w22
        tunnel: [w1174 44100.0 ("Sampling Rate")] -> w95
        tunnel: [w1177 w1192] -> w103
        tunnel: [w1175 w1192] -> w102
        tunnel: [w1172 TRUE] -> w86
        tunnel: [w1171 44100.0 ("Sampling Rate")] -> w30
        frame False {
          w1187 = enum16{"Curves", "Values", "Results", "WFM"}."WFM" ("Type")
          # "response"
          # "stimulus"
          n13 = Unbundle By Name(w1180) -> ("Waveform Out"=w1185:string, "Waveform In"=w1186:string)
          n14 = call "CRYGet Curve Library Data.vi"("Type"=w1187, "Data Name"=w1186) -> ("Wave"=w1189:T7)  [unwired: 4 out]
          n15 = call "CRYGet Curve Library Data.vi"("Type"=w1187, "Data Name"=w1185) -> ("Wave"=w1188:T7)  [unwired: 4 out]
          n16 = Unbundle By Name(w1189) -> ("Waveform.Y"=w1183:sgl[], "Test Info"=w1176:string)
          n17 = Unbundle By Name(w1188) -> ("Waveform.dX"=w1171:dbl, "Waveform.Y"=w1184:sgl[], "Test Info"=w1178:string)
          n18 = call "CRYGet Calibration From Test Infor.vi"("Response Test Information Flatten"=w1176, "Stimulus Test Information Flatten"=w1178) -> ("unflattened Response test infor data"=w1177:T14, "unflattened Stimulus test infor data"=w1175:T14)  [unwired: 5 in, 3 out]
          n19 = Unbundle By Name(w1177) -> ("Signal Type"=w1179:string, "Sampling Rate"=w1174:dbl)
          n20 = Unbundle By Name(w1175) -> ("Sampling Rate"=w1173:dbl)
          n21 = To Double Precision Float(number=w1184) -> (double precision float=w1181:dbl[])
          n22 = To Double Precision Float(number=w1183) -> (double precision float=w1182:dbl[])
          n23 = Equal?(x=w1174, y=w1173) -> (x = y?=w1172:bool)
        }
        frame True {
          w1192 = T14 {"Stimulus Type"="", "Signal Type"="", "In/Out"=FALSE, "FAPS"=[], "Sampling Rate"=0.0, "Samples"=0, "Analysis Param"="", "Resolution"=0, "Steps"=0, "Analysis Value"=[], "Diff Freq"=0.0, "FStart"=0.0, "FStop"=0.0, "Calibration Param"="", "Anti Alias"=0.0, "Level Out1"=0.0, "Level Out2"=0.0, "EQ"=FALSE}  # unflattened test infor cluster
        }
      }
      n24 = Unbundle By Name(w24) -> ("Polarity"=w26:bool, "Imp Ref resistor"=w74:dbl, "Algorithm"=w119:u16, "Imp"=w107:bool, "impulse"=w118:bool, "Deconvolved Response"=w113:bool, "Standard Error"=w73:bool, "Confidence Limits"=w72:bool, "Total Noise"=w71:bool, "Harmonics @ meas.frq"=w70:bool, "Total Distortion"=w69:bool, "THD(%)"=w68:bool, "THD Normalized(%)"=w67:bool, "THD+Noise(%)"=w66:bool, "Rub&Buzz"=w65:bool, "Rub&Buzz Norm'd(%)"=w64:bool, "Perceptual Rub&Buzz"=w31:bool, "Total IM"=w63:bool, "Total IMD(%)"=w62:bool, "Total IMD + Noise(%)"=w61:bool, "Total Diff"=w60:bool, "Total DFD(%)"=w59:bool, "Total DFD+Noise(%)"=w58:bool, "Type"=w53:u16, "Weigting"=w55:string, "TSR Window Type"=w54:string)
      n25 = Unbundle By Name(w24) -> ("delay"=w109:dbl, "Distance Unit"=w104:u16, "Delay Method"=w108:u16, "Use Channel Name"=w19:bool, "Waveform In"=w85:string, "Waveform Out"=w84:string)
      n26 = Unbundle By Name(w24) -> ("Harmonics"=w77:dbl[], "Type"=w80:u16, "Algorithm"=w81:u16, "Intermod"=w78:dbl[], "Diff"=w82:dbl[])
      n27 = case shown="Default" w81 {
        tunnel: w77 -> [w1200 w1204]
        tunnel: w78 -> [w1199 _]
        tunnel: w82 -> [w1198 _]
        tunnel: [w1197 w1204] -> w79
        tunnel: w80 -> [w1196 _]
        frame Default {
          n28 = case shown="0, Default" w1196 {
            tunnel: w1200 -> [w1201 _ _]
            tunnel: [w1201 w1202 w1203] -> w1197
            tunnel: w1199 -> [_ w1202 _]
            tunnel: w1198 -> [_ _ w1203]
            frame 0, Default {
            }
            frame 1 {
            }
            frame 2 {
            }
          }
        }
        frame 4 {
        }
      }
      n29 = Build Array(w73, w72, w71, w70, w69, w68, w67, w66, w65, w64, w31, w63, w62, w61, w60, w59, w58) -> (w52:bool[])
      n30 = local write "Ref resistor"(w74) -> ()
      n31 = call "CRYGet Number to Window.vi"("TSR Window Name"=w54, "Weighting Name"=w55) -> ("TSR window"=→"TSR window":u16, "Weighting"=→"Window":u16)  [unwired: 2 in]
      n32 = call "CRYCheck HT Option.vi"("Option Array In"=w52, "Type"=w53, "Algorithm"=w119) -> ("Option Array Out"=w51:bool[])  [unwired: 8 in]
      "HT Option" <- w51
      n33 = case shown="Default" w81 {
        tunnel: [dbl[] [1.0] ("Harmonics") w128] -> w76
        tunnel: w79 -> [_ w126]
        tunnel: [TRUE ("Make Fundamental curve?") w127] -> w75
        tunnel: w80 -> [_ w125]
        frame Default {
        }
        frame 2, 4 {
          n34 = call "CRYHarmonics array order.vi"("Type"=w125, "Harmonics array in"=w126) -> ("Make Fundamental curve?"=w127:bool, "Harmonics array out"=w128:dbl[])  [unwired: 8 out]
        }
      }
      n35 = case shown="False" w86 {
        tunnel: w85 -> [w131 _]
        tunnel: w84 -> [w130 _]
        frame False {
          n36 = call "CRYGet Error Message.vi"("Error No"=8, "Kind"="Analysis") -> ("Message"=w129:string, "Window Title"=w133:string)  [unwired: 4 in, 4 out]
          n37 = Format Into String(format string=w129, w131, w130) -> (resulting string=w132:string)  [unwired: 2 in, 1 out]
          n38 = call "CRYMessage Dialog.vi"("Window Title"=w133, "Message Content"=w132) -> ()  [unwired: 8 in, 2 out]
        }
        frame True {
        }
      }
      n39 = Reciprocal(x=w95) -> (1/x=w46:dbl)
      n40 = Bundle By Name("Y"=w29, "dt"=w30) -> (→"Stimulus Waveform":waveform(dbl))  [unwired: 1 in]
      n41 = Not Equal?(x=w22, y="") -> (x != y?=w20:bool)
      n42 = Bundle By Name("Y"=w94, "dt"=w46) -> (→"Response Waveform":waveform(dbl))  [unwired: 1 in]
      n43 = And(x=w20, y=w19) -> (x .and. y?=w21:bool)
      n44 = case shown="False" w21 {
        tunnel: w22 -> [_ w153]
        tunnel: ["" w152] -> w112
        frame False {
        }
        frame True {
          n45 = Concatenate Strings(" [" ("string"), w153, "]" ("string")) -> (w152:string)
        }
      }
      "Channel Label In" <- w112
      n46 = case shown="0" w108 {
        tunnel: w95 -> [w1153 w1167]
        tunnel: w29 -> [_ w1169]
        tunnel: w94 -> [w1152 w1168]
        tunnel: [w1150 w1165] -> w114
        tunnel: [w1147 w1155] -> w106
        tunnel: w112 -> [_ w1170]
        tunnel: w104 -> [_ w1166]
        tunnel: w109 -> [w1149 _]
        tunnel: w24 -> [_ w1164]
        tunnel: w26 -> [_ w1154]
        frame Default {
          (unwired) 0.001
          # "Fs * t * 0.001"
          # "??????"
          n47 = Compound Arithmetic op=MULTIPLY(w1153, w1149) -> (w1151:dbl)
          n48 = Array Subset(array=w1152, index=w1151) -> (w1150:dbl[])  [unwired: 1 in]
          n49 = Initialize Array("Datum", 0 ("dimension size")) -> (w1147:T2[])
        }
        frame 0 {
          n50 = Unbundle By Name(w1164) -> ("use custom unit"=w1158:bool, "Custom Curve Names"=w1159:string[], "Custom Curve IDs"=w1160:i32[], "Default Curve Names"=w1161:string[], "Use default"=w1163:bool)
          n51 = Bundle(FALSE, "Check Option"="", "use custom unit"=w1158, "Custom Curve Names"=w1159, "Custom Curve IDs"=w1160, "Default Curve Names"=w1161, "Use default"=w1163) -> (w1162:T15)  [unwired: 1 in]
          n52 = call "CRYAna Auto Delay.vi"("Additive Info"=w1162, "Distance Unit"=w1166, "Polarity"=w1154, "Fs"=w1167, "Response"=w1168, "Stimulus"=w1169, "Channel Name"=w1170) -> ("Result Response"=w1165:dbl[], "Value Out"=w1155:T2[])  [unwired: 2 in, 1 out]
        }
      }
      n53 = stacked-sequence {
        seq-local: [w196 _ _ _ _] -> [_ w317 w591 _ _]
        seq-local: [w195 _ _ _ _] -> [_ w316 _ _ _]
        seq-local: [w194 _ _ _ _] -> [_ w311 w586 _ _]
        seq-local: [_ w297 _ _ _] -> [_ _ w577 _ _]
        seq-local: [w191 _ _ _ _] -> [_ w315 w572 w920 w1087]
        seq-local: [w192 _ _ _ _] -> [_ _ w584 _ _]
        seq-local: [_ w312 _ _ _] -> [_ _ _ w919 _]
        seq-local: [_ _ w583 _ _] -> [_ _ _ w921 _]
        seq-local: [_ _ w566 _ _] -> [_ _ _ w914 _]
        seq-local: [_ w307 _ _ _] -> [_ _ _ _ _]
        seq-local: [w180 _ _ _ _] -> [_ w304 _ _ _]
        seq-local: [w179 _ _ _ _] -> [_ w303 _ _ _]
        tunnel: [_ _ _ w915 _] -> w117
        tunnel: "Manual?" -> [w193 _ _ _ _]
        tunnel: w119 -> [w187 w301 w576 w916 w1101]
        tunnel: w114 -> [_ w299 _ _ _]
        tunnel: w118 -> [_ w314 _ _ _]
        tunnel: w76 -> [_ w296 w582 w917 w1102]
        tunnel: w75 -> [_ _ w573 _ w1100]
        tunnel: w24 -> [w189 w308 w579 w913 w1085]
        tunnel: [_ _ _ _ w1075] -> w115
        tunnel: w113 -> [_ w313 _ _ _]
        tunnel: w29 -> [_ w310 _ _ w1093]
        tunnel: w107 -> [_ _ _ w918 _]
        tunnel: w106 -> [_ _ _ _ w1097]
        tunnel: [_ _ _ _ w1076] -> w105
        tunnel: w94 -> [_ w300 _ _ w1078]
        tunnel: w103 -> [w181 w302 w559 _ w1091]
        tunnel: w102 -> [w182 w305 _ _ w1069]
        tunnel: w51 -> [_ _ _ _ _]
        frame #0 {
          w188 = u16 6  # Transfer
          w190 = 2  # Log amp sweep
          # "Response"
          # "stimulus"
          # "cycle\nfreq\namp"
          n54 = Unbundle By Name(w181) -> ("Calibration Param"=w183:string)
          n55 = Unbundle By Name(w182) -> ("Calibration Param"=w184:string)
          n56 = Unbundle By Name(w182) -> ("Stimulus Type"=w185:string)
          n57 = Equal?(x=w187, y=w188) -> (x = y?=w186:bool)
          n58 = Search 1D Array(1D array=string[] ["Frequency Stepped Sweep", "Frequency Log Sweep", "Log Amplitude Sweep", "WAV", "DC Connect", "Two Tone", "Noise", "Multitone"] ("Strings []"), element=w185) -> (index of element=w178:i32)  [unwired: 1 out]
          n59 = Unflatten From String(type="Calibration All Cluster", binary string=w184) -> (value=w180:T4)  [unwired: 2 in, 3 out]
          n60 = Unflatten From String(type="Calibration All Cluster", binary string=w183) -> (value=w179:T4)  [unwired: 2 in, 3 out]
          n61 = Equal?(x=w178, y=w190) -> (x = y?=w191:bool)
          n62 = case shown="False" w193 {
            tunnel: [w234 w287] -> w195
            tunnel: [w236 "Frequency [Hz]"] -> w196
            tunnel: [w235 w291] -> w194
            tunnel: [w216 1.0 ("dB Ref Out")] -> w192
            tunnel: w189 -> [w215 _]
            tunnel: w186 -> [w214 _]
            tunnel: w182 -> [w211 _]
            tunnel: w181 -> [w212 _]
            tunnel: w180 -> [w208 _]
            tunnel: w179 -> [w209 _]
            tunnel: w178 -> [w207 _]
            frame False {
              # "unit???"
              # "V/Pa => Pa"
              # "VV/V => VV"
              # "????? X unit(log amplitude sweep)==2"
              # "Get In/Out Calibration Data!"
              n63 = Unbundle By Name(w212) -> ("Sampling Rate"=w210:dbl)
              n64 = Unbundle By Name(w211) -> ("FStart"=w213:dbl, "FStop"=w206:dbl)
              n65 = case shown="True" w214 {
                tunnel: [w247 w252] -> w236
                tunnel: [w246 w257] -> w235
                tunnel: [w245 w257] -> w234
                tunnel: w215 -> [_ w258]
                tunnel: w210 -> [_ _]
                tunnel: w213 -> [_ w256]
                tunnel: w211 -> [w244 _]
                tunnel: w207 -> [_ _]
                tunnel: w206 -> [_ w255]
                frame False {
                  n66 = Unbundle By Name(w244) -> ("FAPS"=w243:T16)
                  n67 = for {
                    tunnel: w243 -> [w251] mode=indexing
                    tunnel: [w250] -> w247 mode=indexing
                    tunnel: [w248] -> w246 mode=indexing
                    tunnel: [w249] -> w245 mode=indexing
                    n68 = Unbundle By Name(w251) -> ("freq"=w250:dbl, "ampl"=w248:dbl, "cycles"=w249:dbl)
                  }
                }
                frame True {
                  w257 = dbl[] [1.0]
                  n69 = Unbundle By Name(w258) -> ("Freq.Resolution"=w254:dbl)
                  n70 = while {
                    tunnel: w256 -> [w266]
                    tunnel: w255 -> [w261]
                    tunnel: w254 -> [w267]
                    shift-right: [w263] -> w252
                    shift-left: dbl[] [] ("appended array") -> [w264]
                    i -> [w268]
                    stop <- w259 stop-if-true
                    n71 = Multiply(x=w267, y=w268) -> (x*y=w265:dbl)
                    n72 = Add(x=w266, y=w265) -> (x+y=w260:dbl)
                    n73 = Greater?(x=w260, y=w261) -> (0:w262:bool)
                    n74 = case shown="False" w262 {
                      selector: w262 -> [w270 w273]
                      tunnel: [w271 w274] -> w263
                      tunnel: w264 -> [w272 w274]
                      tunnel: [w270 w273] -> w259
                      tunnel: w260 -> [w269 _]
                      frame False {
                        n75 = Build Array (concatenate)(w272, w269) -> (w271:dbl[])
                      }
                      frame True {
                      }
                    }
                  }
                }
              }
              n76 = Unbundle By Name(w208) -> ("Sens Curve.Curve"=w221:cluster{"x":dbl, "y":dbl, "z":dbl}[], "Sens Curve.Y dB ref"=w216:dbl, "Sens Curve.Y unit"=w233:string)
              "Y dB ref Out" <- w216
              n77 = Unbundle By Name(w209) -> ("Sens Curve.Y dB ref"=w204:dbl, "Sens Curve.Y unit"=w225:string, "Sens Curve.Curve"=w222:cluster{"x":dbl, "y":dbl, "z":dbl}[])
              "Y dB ref In" <- w204
              n78 = Unbundle By Name(w215) -> ("use custom unit"=w203:bool, "Y unit"=w202:string, "Y dB ref"=w201:dbl, "Y data"=w200:u16, "Scaling"=w220:i32)
              n79 = Index Array(array=w222) -> (element=w239:cluster{"x":dbl, "y":dbl, "z":dbl})  [unwired: 1 in]
              n80 = Index Array(array=w221) -> (element=w237:cluster{"x":dbl, "y":dbl, "z":dbl})  [unwired: 1 in]
              n81 = Search/Split String(string=w225, search string/char (-)="/" ("search char (-)")) -> (substring before match=w229:string, match + rest of string=w231:string, offset of match=w227:i32)  [unwired: 1 out]
              n82 = Search/Split String(string=w233, search string/char (-)="/" ("search char (-)")) -> (substring before match=w217:string)  [unwired: 3 out]
              "Y unit Out" <- w217
              n83 = Unbundle By Name(w239) -> ("y"=w238:dbl)
              n84 = Unbundle By Name(w237) -> ("y"=w224:dbl)
              n85 = String Subset(string=w231, offset (0)=1) -> (substring=w232:string)  [unwired: 1 in]
              n86 = Greater Or Equal To 0?(x=w227) -> (x >= 0?=w228:bool)
              n87 = global read "CRYCal Global.vi" "Calibrate"() -> (w242:bool)
              n88 = Select(t=w232, s=w228, f=w229) -> (s? t:f=w205:string)
              "Y unit In" <- w205
              n89 = case shown="False" w203 {
                tunnel: w201 -> [_ w279]
                tunnel: w202 -> [_ w280]
                tunnel: [w276 w280] -> w199
                tunnel: w204 -> [w277 _]
                tunnel: w205 -> [w276 _]
                tunnel: [w277 w279] -> w198
                tunnel: w200 -> [_ w278]
                tunnel: [u16 0 ("Y data") w278] -> w197
                frame False {
                }
                frame True {
                }
              }
              "Y Unit Curve" <- w199
              "Y dB ref Curve" <- w198
              n90 = case shown="True" w242 {
                tunnel: [w281 w284] -> w241
                tunnel: w238 -> [w281 _]
                tunnel: w224 -> [w282 _]
                tunnel: [w282 w283] -> w223
                frame False {
                }
                frame True {
                  n91 = global read "CRYCal Global.vi" "Sens Out"() -> (w283:dbl)
                  n92 = global read "CRYCal Global.vi" "Sens In"() -> (w284:dbl)
                }
              }
              "Sens In" <- w241
              "Sens Out" <- w223
              n93 = local write "Y data Curve"(w197) -> ()
              n94 = To Unsigned Word Integer(number=w220) -> (unsigned 16bit integer=w218:u16)
              n95 = Bundle("Y unit"=w205, "Y dB ref"=w204, "Y unit"=w217, "Y dB ref"=w216, "Y unit"=w199, "Y dB ref"=w198, "Y data"=w197, w218) -> (→"Unit Info":T17)  [unwired: 1 in]
            }
            frame True {
              n96 = Array Size(array="Frequency [Hz]") -> (size(s)=w290:i32)
              n97 = To Double Precision Float(number="cycles") -> (double precision float=w286:dbl)
              n98 = Array Size(array="Frequency [Hz]") -> (size(s)=w293:i32)
              n99 = local write "Y data Curve"(u16 1 ("Y data")) -> ()
              n100 = local write "Sens In"(1.0 ("Sens In")) -> ()
              n101 = Initialize Array(w286, w290) -> (w287:dbl[])
              n102 = Initialize Array(1.0 ("Level left"), w293) -> (w291:dbl[])
            }
          }
        }
        frame #1 {
          n103 = Unbundle By Name(w302) -> ("Sampling Rate"=w298:dbl, "Samples"=w306:i32)
          n104 = local read "Sens In"() -> (w309:dbl)
          n105 = case shown="4" w301 {
            selector: w301 -> [_ _ w369 w438 w497 w524]
            tunnel: w298 -> [w330 w359 w362 w419 w483 w537]
            tunnel: w317 -> [w331 _ w366 _ w494 w544]
            tunnel: w316 -> [w332 _ w367 _ _ w550]
            tunnel: w311 -> [_ _ w365 _ _ w549]
            tunnel: w309 -> [w329 w354 w381 _ _ w538]
            tunnel: w299 -> [w326 w350 w370 w453 w493 _]
            tunnel: w296 -> [_ _ w392 w420 _ w539]
            tunnel: [w322 w347 w375 w430 w491 w525] -> w297
            tunnel: w315 -> [_ _ w397 w418 _ w548]
            tunnel: w308 -> [w325 w361 w393 w461 w501 w540]
            tunnel: w314 -> [_ _ _ _ _ _]
            tunnel: w313 -> [_ _ _ _ _ _]
            tunnel: [T12 [] ("Harmonic Track Out") T12 [] ("Harmonic Track Out") w372 w439 T12 [] ("Harmonic Track Out") _] -> w312
            tunnel: [w326 w350 w370 w453 w493 w536] -> w307
            tunnel: w310 -> [_ _ w371 w436 w499 _]
            tunnel: w303 -> [w320 w343 w376 w448 w487 w535]
            tunnel: w304 -> [w321 w344 w377 w449 w488 w534]
            tunnel: w305 -> [_ w337 w386 w427 w477 w528]
            tunnel: w302 -> [_ _ _ w460 _ _]
            tunnel: w306 -> [_ w349 _ _ _ _]
            tunnel: w300 -> [_ _ _ _ _ w522]
            tunnel: w299 -> [_ _ _ w437 _ w519]
            frame 0 {
              # "BroadBand RMS"
              n106 = Unbundle By Name(w325) -> ("discard cycles"=w324:dbl, "Apply Correction Out"=w319:bool, "Apply Correction In"=w318:bool)
              n107 = Bundle("Sampling Rate"=w330, "discard cycles"=w324, "Sens In"=w329, "AC/DC"="AC/DC") -> (w327:T18)  [unwired: 1 in]
              n108 = call "CRYAna Broadband RMS.vi"("Info"=w327, "Freq"=w331, "Cycles"=w332, "Response"=w326) -> ("Freq resp curves"=w323:cluster{cluster{"Fi":dbl, dbl, dbl}[]}[])  [unwired: 7 in]
              n109 = call "CRYCal Correction.vi"("Calibration Response Cluster"=w320, "Calibration Stimulus Cluster"=w321, "Apply Corr In"=w318, "Apply Corr Out"=w319, "Frequency curve in"=w323) -> ("Frequency curve out"=w322:cluster{cluster{"x":dbl, "y":dbl, "z":dbl}[]}[])  [unwired: 6 in]
            }
            frame 1 {
              # "??????????"
              # "Spectrum"
              n110 = Unbundle By Name(w361) -> ("Freq.Resolution"=w334:dbl, "Overlap"=w355:dbl, "Spectral Scaling"=w351:u16, "Apply Correction Out"=w346:bool, "Apply Correction In"=w345:bool)
              n111 = Unbundle By Name(w337) -> ("Signal Type"=w340:string, "EQ"=w338:bool, "Level Out2"=w335:dbl)
              n112 = local read "Window"() -> (w356:u16)
              n113 = To Double Precision Float(number=w349) -> (double precision float=w357:dbl)
              n114 = call "CRYGet Current Calibration Info.vi"("Is Input?"=FALSE, "Signal Type Name"=w340) -> ("Calibration All Cluster"=w341:T4)  [unwired: 9 out]
              n115 = Bundle("Sampling Rate"=w359, w357) -> (w358:cluster{"Sampling Rate":dbl, dbl})  [unwired: 1 in]
              n116 = Bundle("Window"=w356, "Freq.Resolution"=w334, "Overlap"=w355, "Spectral Scaling"=w351, "Sens In"=w354) -> (w353:T19)  [unwired: 1 in]
              n117 = Unbundle By Name(w341) -> ("EQ Curve"=w339:T2)
              n118 = Bundle("EQ Curve"=w339, "EQ"=w338, "Level Out2"=w335) -> (w336:T20)  [unwired: 1 in]
              n119 = call "CRYAna Spectrum.vi"("EQ information"=w336, "Infor"=w353, "Wave Infor"=w358, "Signal"=w350) -> ("Spectrum X-axis"=→"Spectrum X-axis":dbl[], "Freq resp curves"=w348:cluster{cluster{dbl, dbl, dbl}[]}[])  [unwired: 5 in, 1 out]
              n120 = call "CRYCal Correction.vi"("Calibration Response Cluster"=w343, "Calibration Stimulus Cluster"=w344, "Apply Corr In"=w345, "Apply Corr Out"=w346, "Frequency curve in"=w348) -> ("Frequency curve out"=w347:cluster{cluster{"x":dbl, "y":dbl, "z":dbl}[]}[])  [unwired: 6 in]
            }
            frame 2 {
              # "Harmonic"
              n121 = Unbundle By Name(w393) -> ("Method"=w395:u16, "ResponseMe"=w382:u16, "discard cycles"=w364:dbl, "Type"=w394:u16, "Apply Correction Out"=w389:bool, "Apply Correction In"=w388:bool, "Std Err"=w378:dbl, "Perceptual Rub&Buzz"=w374:bool)
              n122 = Unbundle By Name(w386) -> ("Diff Freq"=w385:dbl, "FAPS"=w368:T16)
              n123 = local read "HT Option"() -> (w396:bool[])
              n124 = local read "Window"() -> (w363:u16)
              n125 = Less Or Equal?(x=w369, y=u16 1 ("Algorithm")) -> (x <= y?=w391:bool)
              n126 = Compound Arithmetic op=AND(invert w391, w389) -> (w390:bool)
              n127 = Bundle("ResponseMe"=w382, "Sampling Rate"=w362, "Sens In"=w381) -> (w383:T21)  [unwired: 1 in]
              n128 = Bundle("Window"=w363, "discard cycles"=w364) -> (w384:cluster{"Window":u16, "discard cycles":dbl})  [unwired: 1 in]
              n129 = Bundle(w367, "Frequency [Hz]"=w366, w365, w397, "Diff Freq"=w385) -> (w380:T22)  [unwired: 1 in]
              n130 = Bundle("Type"=w394, "Method"=w395, "HT Option"=w396, "Harmonics array out"=w392, w390, "Apply Correction In"=w388, "Std Err"=w378) -> (w379:T23)  [unwired: 1 in]
              n131 = call "CRYAna Harmonic.vi"("Calibration Response Cluster"=w376, "Distortion Infor"=w379, "Calibration Stimulus Cluster"=w377, "Stimulus Infor"=w380, "Time Infor"=w384, "Wave Infor"=w383, "Response"=w370, "Algorithm"=w369) -> ("Freq resp curves clipped"=w375:cluster{cluster{"x":dbl, "y":dbl, "z":dbl}[]}[], "Harmonic Track Out"=w373:T12)  [unwired: 2 in]
              n132 = case shown="True" w374 {
                tunnel: w373 -> [w398 w412]
                tunnel: [w398 w411] -> w372
                tunnel: w371 -> [_ w410]
                tunnel: w370 -> [_ w409]
                tunnel: w369 -> [_ w408]
                tunnel: w368 -> [_ w407]
                tunnel: w367 -> [_ w405]
                tunnel: w366 -> [_ w404]
                tunnel: w365 -> [_ w403]
                tunnel: w364 -> [_ w402]
                tunnel: w363 -> [_ w401]
                tunnel: w362 -> [_ w400]
                frame False {
                }
                frame True {
                  n133 = for {
                    tunnel: [w414] -> w406 mode=indexing
                    tunnel: w407 -> [w413] mode=indexing
                    n134 = Unbundle By Name(w413) -> ("samples"=w414:i32)
                  }
                  n135 = Bundle(w405, "Frequency [Hz]"=w404, w403, w406, "Sampling Rate"=w400, "Window"=w401, "discard cycles"=w402) -> (w399:T24)  [unwired: 1 in]
                  n136 = call "CRYAna Perceptual Rub&Buzz.vi"("Harmonic Infor"=w399, "Harmonic Track In"=w412, "Response"=w409, "Stimulus"=w410, "Algorithm"=w408) -> ("Harmonic Track Out"=w411:T12)  [unwired: 6 in]
                }
              }
            }
            frame 4 {
              w459 = T25 {"FSamp"=0.0, "FStart"=0.0, "FStop"=0.0, "NOffset"=0.0, "MStop"=0.0, "MStart"=0.0, "NHarm"=0.0, "Tsamp"=0.0, "Amplit"=0.0, "Amplit 2"=0.0}  # TSR params
              # "Time Selective Response"
              # "TSR"
              n137 = Unbundle By Name(w427) -> ("Signal Type"=w426:string, "EQ"=w424:bool, "Level Out2"=w422:dbl)
              n138 = call "CRYGet Current Calibration Info.vi"("Is Input?"=FALSE, "Signal Type Name"=w426) -> ("Calibration All Cluster"=w428:T4)  [unwired: 9 out]
              n139 = Unbundle By Name(w428) -> ("EQ Curve"=w425:T2)
              n140 = Bundle("EQ Curve"=w425, "EQ"=w424, "Level Out2"=w422) -> (w423:T20)  [unwired: 1 in]
              n141 = Unbundle By Name(w461) -> ("Method"=w417:u16, "Apply Correction Out"=w451:bool, "Apply Correction In"=w450:bool, "TSR Window Type"=w447:string, "start ms"=w446:dbl, "stop ms"=w445:dbl, "Over-samples Res."=w444:dbl, "ResponseMe"=w443:u16, "Scaling"=w442:i32, "Perceptual Rub&Buzz"=w441:bool, "Curve Resolution"=w434:u16, "Curve Resolution Hz"=w433:dbl, "Std Err"=w431:dbl)
              n142 = Unbundle By Name(w460) -> ("Analysis Param"=w454:string)
              n143 = Bundle("TSR Window Type"=w447, "start ms"=w446, "stop ms"=w445, "Over-samples Res."=w444) -> (w458:T26)  [unwired: 1 in]
              n144 = Unflatten From String(type=w459, binary string=w454) -> (value=w435:T25)  [unwired: 1 in, 4 out]
              n145 = call "CRYAna TSR.vi"("Response"=w437, "Abs/Rel"=w443, "dz(Hz)"=w433, "EQ information"=w423, "Harmonics"=w420, "Parameter In"=w458, "Resolution"=w434, "TSR params"=w435, "Stimulus"=w436, "Impulse data type(db/Lin)"=w442) -> ("Freq resp curves"=w452:cluster{cluster{"x":dbl, "y":dbl, "z":dbl}[]}[], "X axis, fundamental"=w457:dbl[], "Total Noise"=w416:dbl[], "Impulse response"=→"Impulse Resp Y":dbl[][], "Impulse time axis"=→"Impulse Resp X":dbl[])  [unwired: 1 out]
              n146 = local write "Spectrum X-axis"(w457) -> ()
              n147 = call "CRYCal Correction.vi"("Calibration Response Cluster"=w448, "Calibration Stimulus Cluster"=w449, "Apply Corr In"=w450, "Apply Corr Out"=w451, "Frequency curve in"=w452) -> ("Frequency curve out"=w432:cluster{cluster{"x":dbl, "y":dbl, "z":dbl}[]}[])  [unwired: 6 in]
              n148 = local read "HT Option"() -> (w415:bool[])
              n149 = call "CRYharmonic curves clipf.vi"("Fs"=w419, "Harmonics"=w420, "Freq resp curves"=w432) -> ("Freq resp curves clipped"=w421:cluster{cluster{"x":dbl, "y":dbl, "z":dbl}[]}[])  [unwired: 8 out]
              n150 = call "CRYAlignment Harmonic curves.vi"("Harmonics order"=w420, "HT Option"=w415, "Std Error"=w431, "Harmonic Curves"=w421) -> ("Freq Curves Out"=w430:cluster{cluster{"x":dbl, "y":dbl, "z":dbl}[]}[])  [unwired: 7 in]
              n151 = call "CRYCalc Rub Buzz for PRB.vi"("Total Noise"=w416, "HT Option"=w415, "Method"=w417, "Amplitude sweep (F)"=w418, "Fs"=w419, "Harmonics"=w420, "Freq resp curves"=w421) -> ()  [unwired: 2 in, 3 out]
              n152 = call "CRYCalc Rub Buzz THD.vi"("Total Noise"=w416, "HT Option"=w415, "Method"=w417, "Amplitude sweep (F)"=w418, "Fs"=w419, "Harmonics"=w420, "Freq resp curves"=w421) -> ("Harmonic Track Out"=w440:T12)  [unwired: 4 out]
              n153 = case shown="True" w441 {
                tunnel: w440 -> [w462 w474]
                tunnel: [w462 w473] -> w439
                tunnel: w438 -> [_ w472]
                tunnel: w437 -> [_ w471]
                tunnel: w436 -> [_ w470]
                tunnel: w435 -> [_ w469]
                tunnel: w419 -> [_ w467]
                frame False {
                }
                frame True {
                  w465 = dbl[] []
                  n154 = Bundle(w465, w465, w465, i32[] [], "Sampling Rate"=w467, "Window"=u16 0, "Sampling Rate"=0.0) -> (w468:T27)  [unwired: 1 in]
                  n155 = call "CRYAna Perceptual Rub&Buzz.vi"("TSR params"=w469, "Harmonic Infor"=w468, "Harmonic Track In"=w474, "Response"=w471, "Stimulus"=w470, "Algorithm"=w472) -> ("Harmonic Track Out"=w473:T12)  [unwired: 5 in]
                }
              }
            }
            frame 5, 6 {
              n156 = Unbundle By Name(w477) -> ("Signal Type"=w480:string, "EQ"=w478:bool, "Level Out2"=w475:dbl)
              n157 = Unbundle By Name(w501) -> ("ResponseMe"=w486:u16, "Auto Spectrum(Stimulus)*"=w517:bool, "Auto Spectrum(Response)*"=w516:bool, "Cross Spectrum*"=w515:bool, "Coherent Power*"=w514:bool, "Non-Coherent Power*"=w513:bool, "Frequency Response"=w512:bool, "Coherence (%)"=w511:bool, "Non-Coherence (%)"=w510:bool, "Signal-Noise Ratio (dB)"=w509:bool, "Non-Coherenct Distirtion*"=w508:bool, "Averaging"=w496:u16, "Spectral Scaling"=w503:u16, "Curve Resolution Hz"=w507:dbl, "Overlap"=w506:dbl, "Apply Correction Out"=w490:bool, "Apply Correction In"=w489:bool)
              n158 = Unbundle By Name(w477) -> ("Level Out1"=w484:dbl)
              n159 = local read "Window"() -> (w505:u16)
              n160 = call "CRYGet Current Calibration Info.vi"("Is Input?"=FALSE, "Signal Type Name"=w480) -> ("Calibration All Cluster"=w481:T4)  [unwired: 9 out]
              n161 = Unbundle By Name(w481) -> ("EQ Curve"=w479:T2)
              n162 = Bundle("Curve Resolution Hz"=w507, "Overlap"=w506, "Window"=w505) -> (w504:T28)  [unwired: 1 in]
              n163 = Bundle("Averaging"=w496, "Spectral Scaling"=w503) -> (w502:cluster{"Averaging":u16, "Spectral Scaling":u16})  [unwired: 1 in]
              n164 = Build Array(w517, w516, w515, w514, w513, w512, w511, w510, w509, w508) -> (w498:bool[])
              n165 = Bundle("EQ Curve"=w479, "EQ"=w478, "Level Out2"=w475) -> (w476:T20)  [unwired: 1 in]
              n166 = call "CRYCheck Freq Option.vi"("Option Array In"=w498, "Averaging"=w496, "Algorithm"=w497) -> ("Option Array Out"=w495:bool[])  [unwired: 8 in]
              "Freq Option" <- w495
              n167 = Bundle("Sampling Rate"=w483, "Level Out1"=w484) -> (w485:cluster{"Sampling Rate":dbl, "Level Out1":dbl})  [unwired: 1 in]
              n168 = call "CRYAna Frequency.vi"("Option In"=w495, "Abs/Rel"=w486, "Stimulus Infor"=w485, "Stimulus"=w499, "Response"=w493, "Option"=w502, "Freq"=w494, "Time cluster"=w504, "EQ information"=w476) -> ("Curve Out"=w492:cluster{cluster{"cycles":dbl, dbl, dbl}[]}[])  [unwired: 6 in]
              n169 = call "CRYCal Correction.vi"("Calibration Response Cluster"=w487, "Calibration Stimulus Cluster"=w488, "Apply Corr In"=w489, "Apply Corr Out"=w490, "Frequency curve in"=w492) -> ("Frequency curve out"=w491:cluster{cluster{"x":dbl, "y":dbl, "z":dbl}[]}[])  [unwired: 6 in]
            }
            frame 3, Default {
              # "Heterodyne"
              n170 = global read "CRYCal Global.vi" "SoundCard Calibrate"() -> (w523:bool)
              n171 = global read "CRYCal Global.vi" "SoundCard CRY6181"() -> (w521:bool)
              n172 = Unbundle By Name(w540) -> ("Method"=w543:u16, "ResponseMe"=w554:u16, "discard cycles"=w542:dbl, "Type"=w541:u16, "Apply Correction Out"=w531:bool, "Apply Correction In"=w530:bool, "Std Err"=w526:dbl)
              n173 = local read "HT Option"() -> (w546:bool[])
              n174 = Unbundle By Name(w528) -> ("Diff Freq"=w527:dbl)
              n175 = local read "Window"() -> (w552:u16)
              n176 = Less Or Equal?(x=w524, y=u16 1 ("Algorithm")) -> (x <= y?=w533:bool)
              n177 = Compound Arithmetic op=AND(invert w533, w531) -> (w532:bool)
              n178 = Select(t=w522, s=w523, f=w519) -> (s? t:f=w520:dbl[])
              n179 = Bundle("Window"=w552, "discard cycles"=w542) -> (w551:cluster{"Window":u16, "discard cycles":dbl})  [unwired: 1 in]
              n180 = Bundle("ResponseMe"=w554, "Sampling Rate"=w537, "Sens In"=w538) -> (w553:T21)  [unwired: 1 in]
              n181 = Bundle(w550, "Frequency [Hz]"=w544, w549, w548, "Diff Freq"=w527) -> (w547:T22)  [unwired: 1 in]
              n182 = Bundle("Type"=w541, "Method"=w543, "HT Option"=w546, "Harmonics array out"=w539, w532, "Apply Correction In"=w530, "Std Err"=w526) -> (w545:T23)  [unwired: 1 in]
              n183 = Select(t=w519, s=w521, f=w520) -> (s? t:f=w518:dbl[])
              n184 = call "CRYAna Hetero.vi"("Calibration Response Cluster"=w535, "Distortion Infor"=w545, "Calibration Stimulus Cluster"=w534, "Stimulus Infor"=w547, "Time Infor"=w551, "Wave Infor"=w553, "Response"=w518, "Algorithm"=w524) -> ("Freq resp curves clipped"=w525:cluster{cluster{"x":dbl, "y":dbl, "z":dbl}[]}[], "Corrected Response Out"=w536:dbl[])  [unwired: 2 in]
            }
          }
        }
        frame #2 {
          # "?????"
          n185 = Unbundle By Name(w559) -> ("Signal Type"=w558:string)
          n186 = Unbundle By Name(w579) -> ("Imp Auto Mode"=w562:u16, "Mic Auto Mode"=w561:u16, "Mic Ref resistor"=w563:dbl, "Imp"=w557:bool, "Spectral Scaling"=w574:u16, "Type"=w578:u16, "Mic Current"=w556:bool, "use custom unit"=w571:bool, "Custom Curve Names"=w570:string[], "Custom Curve IDs"=w569:i32[], "Default Curve Names"=w568:string[], "Use default"=w567:bool)
          n187 = case shown="True" w572 {
            tunnel: w591 -> [w900 _]
            tunnel: w586 -> [_ w901]
            tunnel: [w900 w901] -> w590
            frame False {
            }
            frame True {
              # "ampl. sweep"
            }
          }
          n188 = Or(x=w557, y=w556) -> (x .or. y?=w564:bool)
          n189 = Select(t=w562, s=w557, f=w561) -> (s? t:f=w560:u16)
          n190 = case shown="Default" w576 {
            tunnel: w564 -> [_ w875]
            tunnel: w577 -> [w868 w874]
            tunnel: [w868 w873] -> w585
            tunnel: w557 -> [_ w872]
            tunnel: w563 -> [_ w871]
            tunnel: w560 -> [_ w870]
            tunnel: w558 -> [_ w869]
            frame 1 {
            }
            frame Default {
              n191 = case shown="True" w875 {
                tunnel: w874 -> [w876 w883]
                tunnel: [w876 w881] -> w873
                tunnel: w872 -> [_ w880]
                tunnel: w871 -> [_ w879]
                tunnel: w870 -> [_ w878]
                tunnel: w869 -> [_ w877]
                frame False {
                }
                frame True {
                  n192 = call "CRYCalc Impedance Mic Current.vi"("Signal Type Input Name"=w877, "Auto Mode"=w878, "Mic Ref resistor"=w879, "Impedance"=w880, "Resistor value(Rref)"="Ref resistor", "Freq resp curves(Vref)"=w883) -> ("Freq resp curves out"=w881:cluster{cluster{"x":dbl, "y":dbl, "z":dbl}[]}[])  [unwired: 5 in]
                }
              }
            }
          }
          n193 = case "X settings" shown="True" w572 {
            tunnel: [u16 1 ("Y data") w898] -> w589
            tunnel: [1.0 ("X dB ref") w897] -> w588
            tunnel: [u16 0 ("X axis") w899] -> _
            tunnel: w584 -> [_ w897]
            frame False {
            }
            frame True {
              w898 = u16 0  # dB
              w899 = u16 1  # Lin
              # "ampl. sweep"
            }
          }
          n194 = case shown="Default" w578 {
            tunnel: w582 -> [w865 w866]
            tunnel: [w865 w866] -> w581
            tunnel: [1 ("Array Index") 2 ("Array Index")] -> w580
            frame Default {
            }
            frame 1, 2 {
            }
          }
          n195 = case shown="Default" w576 {
            tunnel: w590 -> [w906 _]
            tunnel: [w906 w912] -> w587
            tunnel: w572 -> [w905 _]
            tunnel: w586 -> [w904 _]
            tunnel: w585 -> [w903 w911]
            tunnel: [w902 w911] -> w565
            frame 2, 3 {
              n196 = case shown="True" w905 {
                tunnel: w904 -> [_ w910]
                tunnel: w903 -> [w907 w909]
                tunnel: [w907 w908] -> w902
                frame False {
                }
                frame True {
                  # "ampl. sweep"
                  n197 = call "CRYHarmonic curves x-axis replace.vi"("New X axis"=w910, "Freq resp curves"=w909) -> ("Freq resp curves out"=w908:cluster{cluster{"x":dbl, "y":dbl, "z":dbl}[]}[])  [unwired: 9 out]
                }
              }
            }
            frame Default {
              n198 = local read "Spectrum X-axis"() -> (w912:dbl[])
            }
          }
          n199 = for {
            tunnel: w587 -> [w886] mode=indexing
            tunnel: w588 -> [w887]
            tunnel: [w885] -> w583 mode=indexing
            tunnel: w589 -> [w884]
            n200 = case shown="..0" w884 {
              tunnel: w886 -> [w890 w893]
              tunnel: w887 -> [w889 _]
              tunnel: [w888 w891] -> w885
              frame ..0 {
                n201 = call "CRYConversion dB-Lin.vi"("dB ref."=w889, "Lin In"=w890) -> ("Log Out"=w888:dbl)  [unwired: 4 in, 3 out]
              }
              frame 1.. {
                n202 = call "CRYUnit Prefix to Multiplier.vi"() -> ("multiplier"=w892:dbl)  [unwired: 1 in, 4 out]
                n203 = Divide(x=w893, y=w892) -> (x/y=w891:dbl)
              }
            }
          }
          n204 = local read "Unit Info"() -> (w575:T6)
          n205 = Build Array(w557, w556) -> (w555:bool[])
          n206 = case shown="5, 6" w576 {
            selector: w576 -> [w606 _]
            tunnel: w573 -> [w610 _]
            tunnel: [w609 w791] -> w566
            tunnel: w565 -> [w594 w789]
            tunnel: w581 -> [w596 _]
            tunnel: w580 -> [w608 _]
            tunnel: w578 -> [w607 _]
            tunnel: w575 -> [w605 w781]
            tunnel: w574 -> [_ w780]
            tunnel: w572 -> [w604 _]
            tunnel: w571 -> [w602 _]
            tunnel: w570 -> [w601 w775]
            tunnel: w569 -> [w600 w776]
            tunnel: w568 -> [w599 w777]
            tunnel: w567 -> [w598 w778]
            tunnel: w555 -> [w592 w771]
            frame Default {
              w595 = T2 {"Name"="", "Curve"=[], "X data"=1, "Y data"=1, "Z data"=1, "X axis"=0, "Y axis"=1, "Z axis"=1, "X unit"="", "Y unit"="", "Z unit"="", "X dB ref"=1.0, "Y dB ref"=1.0, "Z dB ref"=1.0, "single val"=FALSE, "protected"=FALSE, "display X"=TRUE, "display Y"=FALSE, "display Z"=TRUE, "Test Info"="", "Step No."=0, "Plot Settings"={"Color"=0, "Interpolation"=0, "Point Style"=0, "Line Style"=0, "Point Color"=0, "Line Width"=0, "Bar Plot Style"=0, "Fill To"=0}, "AutoProtect"=FALSE}  # Datum
              # "Distortion"
              n207 = case shown="2" w606 {
                tunnel: w607 -> [_ _ _ w652 _ _]
                tunnel: [_ w623 w635 w651 w664 w681] -> w597
                tunnel: w596 -> [_ _ _ w649 _ w679]
                tunnel: w605 -> [_ w622 w636 w650 w665 w680]
                tunnel: [_ w624 w634 w648 w663 w678] -> w593
                tunnel: w604 -> [_ w621 w633 w646 w662 w675]
                tunnel: [_ w619 w631 w643 w660 w673] -> w603
                tunnel: w602 -> [_ w617 w629 w642 w658 w672]
                tunnel: w601 -> [_ w616 w628 w641 w657 w671]
                tunnel: w600 -> [_ w615 w627 w640 w656 w670]
                tunnel: w599 -> [_ w614 w626 w639 w655 w669]
                tunnel: w598 -> [_ w613 w625 w638 w654 w668]
                tunnel: w592 -> [_ w612 _ w637 w653 w666]
                frame Default {
                }
                frame 0 {
                  n208 = Bundle(w621, "Check Option"="", "use custom unit"=w617, "Custom Curve Names"=w616, "Custom Curve IDs"=w615, "Default Curve Names"=w614, "Use default"=w613) -> (w620:T15)  [unwired: 1 in]
                  n209 = call "CRYGet BroadBand Curve.vi"("Unit Info In"=w622, "Additive Info"=w620, "Impedance and Mic Current In"=w612) -> ("Display Array"=w619:T29, "Unit Info Out"=w624:T30[], "Curve Info Array Out"=w623:T31)  [unwired: 6 in]
                }
                frame 1 {
                  n210 = Bundle(w633, "Check Option"="", "use custom unit"=w629, "Custom Curve Names"=w628, "Custom Curve IDs"=w627, "Default Curve Names"=w626, "Use default"=w625) -> (w632:T15)  [unwired: 1 in]
                  n211 = call "CRYGet Spectrum Curve.vi"("Unit Info In"=w636, "Additive Info"=w632) -> ("Display Array"=w631:T29, "Unit Info Out"=w634:T30[], "Curve Info Array Out"=w635:T31)  [unwired: 7 in]
                }
                frame 2 {
                  n212 = local read "HT Option"() -> (w647:bool[])
                  n213 = Bundle(w646, "Check Option"="Dependence Order", "use custom unit"=w642, "Custom Curve Names"=w641, "Custom Curve IDs"=w640, "Default Curve Names"=w639, "Use default"=w638) -> (w644:T15)  [unwired: 1 in]
                  n214 = call "CRYGet Harmonics Curve array.vi"("Impedance and Mic Current In"=w637, "Additive Info"=w644, "Option Array In"=w647, "Unit Info"=w650, "Diff array"=w649, "IM array"=w649, "Harmonics array"=w649, "Type"=w652) -> ("Display Array"=w643:T29, "Unit Info Out"=w648:T30[], "Curve Info Array Out"=w651:T31)  [unwired: 1 out]
                }
                frame 3 {
                  n215 = Bundle(w662, "Check Option"="", "use custom unit"=w658, "Custom Curve Names"=w657, "Custom Curve IDs"=w656, "Default Curve Names"=w655, "Use default"=w654) -> (w661:T15)  [unwired: 1 in]
                  n216 = call "CRYGet Heterodyne Curve.vi"("Unit Info In"=w665, "Additive Info"=w661, "Impedance and Mic Current In"=w653) -> ("Display Array"=w660:T29, "Unit Info Out"=w663:T30[], "Curve Info Array Out"=w664:T31)  [unwired: 6 in]
                }
                frame 4 {
                  n217 = Bundle(w675, "Check Option"="Dependence Order For TSR", "use custom unit"=w672, "Custom Curve Names"=w671, "Custom Curve IDs"=w670, "Default Curve Names"=w669, "Use default"=w668) -> (w667:T15)  [unwired: 1 in]
                  n218 = local read "HT Option"() -> (w676:bool[])
                  n219 = call "CRYGet Harmonics Curve array.vi"("Impedance and Mic Current In"=w666, "Additive Info"=w667, "Option Array In"=w676, "Unit Info"=w680, "Harmonics array"=w679, "Type"=u16 0) -> ("Display Array"=w673:T29, "Unit Info Out"=w678:T30[], "Curve Info Array Out"=w681:T31)  [unwired: 2 in, 1 out]
                }
              }
              n220 = for {
                tunnel: [w703] -> w611 mode=indexing
                tunnel: w594 -> [w702] mode=indexing
                tunnel: w610 -> [w700]
                tunnel: w597 -> [w686] mode=indexing
                tunnel: w593 -> [w697] mode=indexing
                tunnel: w603 -> [w696] mode=indexing
                tunnel: w595 -> [w688]
                i -> [w698]
                n221 = Unbundle By Name(w697) -> ("X unit"=w693:string, "X data"=w695:u16, "Y unit"=w692:string, "Y data Time"=w694:u16, "X axis"=w689:u16, "X dB ref"=w690:dbl, "Y dB ref"=w691:dbl, "single/curve"=w687:bool)  [unwired: 1 out]
                n222 = Equal To 0?(x=w698) -> (x = 0?=w701:bool)
                n223 = Compound Arithmetic op=OR(w700, invert w701) -> (w699:bool)
                n224 = case shown="True" w699 {
                  tunnel: [w718 w744] -> w703
                  tunnel: w692 -> [w717 w735]
                  tunnel: w691 -> [w716 w725]
                  tunnel: w693 -> [w713 w740]
                  tunnel: w689 -> [w712 w728]
                  tunnel: w694 -> [w711 w739]
                  tunnel: w695 -> [w710 w738]
                  tunnel: w690 -> [w709 w737]
                  tunnel: w702 -> [_ w736]
                  tunnel: w696 -> [_ w730]
                  tunnel: w688 -> [w704 w723]
                  tunnel: w687 -> [_ w721]
                  tunnel: w686 -> [_ w720]
                  frame False {
                    w706 = TRUE ("display X")
                    w714 = u16 1 ("Y data")
                    n225 = Bundle By Name(cluster=w704, "Name"="unknown", "single val"=FALSE, "Y unit"=w717, "X data"=w710, "Y data"=w711, "Z data"=w714, "X axis"=w712, "Y axis"=w714, "Z axis"=w714, "X unit"=w713, "Z unit"="deg.", "X dB ref"=w709, "Y dB ref"=w716, "Z dB ref"=1.0 ("X dB ref"), "display X"=w706, "display Y"=w706, "display Z"=w706) -> (w718:T2)
                  }
                  frame True {
                    w741 = u16 1 ("Y data")
                    n226 = Unbundle By Name(w720) -> ("Custom Curve Name"=w719:string)
                    n227 = Unbundle(w736) -> (w727:cluster{"x":dbl, "y":dbl, "z":dbl}[])
                    n228 = Multiply(x=1e-50 ("Y dB ref"), y=w725) -> (x*y=w724:dbl)
                    n229 = for {
                      tunnel: w727 -> [w753] mode=indexing
                      tunnel: w725 -> [w755]
                      tunnel: [w754] -> w729 mode=indexing
                      tunnel: w739 -> [w747]
                      tunnel: w738 -> [w751]
                      tunnel: w737 -> [w750]
                      tunnel: w724 -> [w745]
                      n230 = Unbundle(w753) -> ("x"=w749:dbl, "y"=w756:dbl, "z"=w752:dbl)
                      n231 = case shown="..0" w747 {
                        tunnel: w756 -> [w765 w769]
                        tunnel: w755 -> [w768 _]
                        tunnel: [w767 w769] -> w746
                        tunnel: w745 -> [w764 _]
                        frame ..0 {
                          n232 = Less Or Equal To 0?(x=w765) -> (x <= 0?=w766:bool)
                          n233 = Select(t=w764, s=w766, f=w765) -> (s? t:f=w763:dbl)
                          n234 = call "CRYConversion dB-Lin.vi"("dB ref."=w768, "Lin In"=w763) -> ("Log Out"=w767:dbl)  [unwired: 4 in, 3 out]
                        }
                        frame 1.. {
                        }
                      }
                      n235 = case shown="..0" w751 {
                        tunnel: w749 -> [w759 w760]
                        tunnel: w750 -> [w758 _]
                        tunnel: [w757 w760] -> w748
                        frame ..0 {
                          n236 = call "CRYConversion dB-Lin.vi"("dB ref."=w758, "Lin In"=w759) -> ("Log Out"=w757:dbl)  [unwired: 4 in, 3 out]
                        }
                        frame 1.. {
                          n237 = disable-structure shown="Disabled" {
                            disable-tunnel: w760 -> [w761 _]
                            frame Disabled {
                              n238 = call "CRYUnit Prefix to Multiplier.vi"() -> ("multiplier"=w762:dbl)  [unwired: 1 in, 4 out]
                              n239 = Divide(x=w761, y=w762) -> ()  [unwired: 1 out]
                            }
                            frame Enabled {
                            }
                          }
                        }
                      }
                      n240 = Bundle("x"=w748, "y"=w746, "z"=w752) -> (w754:cluster{"x":dbl, "y":dbl, "z":dbl})  [unwired: 1 out]
                    }
                    n241 = Unbundle By Name(w730) -> ("display X"=w732:bool, "display Y"=w733:bool, "display Z"=w734:bool)
                    n242 = local read "Channel Label In"() -> (w722:string)
                    n243 = Concatenate Strings(w719, w722) -> (w731:string)
                    n244 = Bundle By Name(cluster=w723, "single val"=w721, "Name"=w731, "Curve"=w729, "X data"=w738, "Y data"=w739, "Z data"=w741, "X axis"=w728, "Y axis"=w741, "Z axis"=w741, "X unit"=w740, "Y unit"=w735, "Z unit"="deg.", "X dB ref"=w737, "Y dB ref"=w725, "Z dB ref"=1.0 ("X dB ref"), "display X"=w732, "display Y"=w733, "display Z"=w734) -> (w744:T2)
                  }
                }
              }
              n245 = case shown="False" w610 {
                tunnel: [w683 w685] -> w609
                tunnel: w611 -> [w684 w685]
                tunnel: w608 -> [w682 _]
                frame False {
                  n246 = Array Subset(array=w684, index=w682) -> (w683:T2[])  [unwired: 1 in]
                }
                frame True {
                }
              }
            }
            frame 5, 6 {
              w773 = FALSE
              w787 = T2[] []  # Frequency response
              # "Frequency"
              n247 = local read "Freq Option"() -> (w786:bool[])
              n248 = local read "Channel Label In"() -> (w783:string)
              n249 = Or Array Elements(Boolean array=w771) -> (logical OR=w770:bool)
              n250 = Bundle(w773, "Check Option"="", w773, "Custom Curve Names"=w775, "Custom Curve IDs"=w776, "Default Curve Names"=w777, "Use default"=w778) -> (w772:T32)  [unwired: 1 in]
              n251 = call "CRYGet Frequency Curve array.vi"("Additive Info"=w772, "Spectral Scaling"=w780, "Unit Info In"=w781, "Option Array In"=w786) -> ("Display Array"=w784:T29, "Unit Info Out"=w785:T30[], "Curve Info Array Out"=w779:T31)  [unwired: 5 in]
              n252 = for {
                tunnel: w779 -> [w793] mode=indexing
                tunnel: w783 -> [w795]
                tunnel: [w794] -> w782 mode=indexing
                n253 = Unbundle By Name(w793) -> ("Custom Curve Name"=w792:string)
                n254 = Concatenate Strings(w792, w795) -> (w794:string)
              }
              n255 = call "CRYUnflatten Data.vi"() -> ("Datum"=w790:T2)  [unwired: 1 in, 10 out]
              n256 = for {
                tunnel: w790 -> [w806]
                tunnel: w789 -> [w804]
                tunnel: w786 -> [w801] mode=indexing
                shift-right: [w807] -> w791
                shift-left: w787 -> [w805]
                shift-right: [w803] -> _
                shift-left: 0 -> [w802]
                tunnel: w770 -> [w799]
                tunnel: w782 -> [w798]
                tunnel: w785 -> [w797]
                tunnel: w784 -> [w796]
                n257 = Compound Arithmetic op=AND(w801, invert w799) -> (w800:bool)
                n258 = case shown="True" w800 {
                  tunnel: [w809 w840] -> w807
                  tunnel: w806 -> [_ w835]
                  tunnel: w804 -> [_ w838]
                  tunnel: w805 -> [w809 w839]
                  tunnel: w802 -> [w808 w829]
                  tunnel: [w808 w836] -> w803
                  tunnel: w798 -> [_ w832]
                  tunnel: w797 -> [_ w831]
                  tunnel: w796 -> [_ w830]
                  frame False {
                  }
                  frame True {
                    w821 = u16 1 ("Y data")
                    n259 = Increment(x=w829) -> (x+1=w836:i32)
                    n260 = Index Array(array=w838, index=w829) -> (element=w837:cluster{cluster{"x":dbl, "y":dbl, "z":dbl}[]})
                    n261 = Unbundle(w837) -> (w811:cluster{"x":dbl, "y":dbl, "z":dbl}[])
                    n262 = Index Array(array=w832, index=w829) -> (element=w828:string)
                    n263 = Index Array(array=w831, index=w829) -> (element=w826:T30)
                    n264 = Index Array(array=w830, index=w829) -> (element=w827:T33)
                    n265 = Unbundle By Name(w826) -> ("X dB ref"=w812:dbl, "Y dB ref"=w813:dbl)
                    n266 = Unbundle By Name(w826) -> ("X unit"=w819:string, "X data"=w814:u16, "Y unit"=w818:string, "Y data Time"=w815:u16, "Z unit"=w817:string, "X data"=w816:u16, "single/curve"=w810:bool)
                    n267 = for {
                      tunnel: w811 -> [w849] mode=indexing
                      tunnel: w813 -> [w851]
                      tunnel: [w850] -> w833 mode=indexing
                      tunnel: w815 -> [w847]
                      tunnel: w814 -> [w846]
                      tunnel: w812 -> [w845]
                      n268 = Unbundle(w849) -> ("x"=w843:dbl, "y"=w842:dbl, "z"=w848:dbl)
                      n269 = case shown="1.." w846 {
                        tunnel: w843 -> [w854 w857]
                        tunnel: w845 -> [w853 _]
                        tunnel: [w852 w855] -> w844
                        frame ..0 {
                          n270 = call "CRYConversion dB-Lin.vi"("dB ref."=w853, "Lin In"=w854) -> ("Log Out"=w852:dbl)  [unwired: 4 in, 3 out]
                        }
                        frame 1.. {
                          n271 = call "CRYUnit Prefix to Multiplier.vi"() -> ("multiplier"=w856:dbl)  [unwired: 1 in, 4 out]
                          n272 = Divide(x=w857, y=w856) -> (x/y=w855:dbl)
                        }
                      }
                      n273 = case shown="..0" w847 {
                        tunnel: w842 -> [w860 w863]
                        tunnel: w851 -> [w859 _]
                        tunnel: [w858 w861] -> w841
                        frame ..0 {
                          n274 = call "CRYConversion dB-Lin.vi"("dB ref."=w859, "Lin In"=w860) -> ("Log Out"=w858:dbl)  [unwired: 4 in, 3 out]
                        }
                        frame 1.. {
                          n275 = call "CRYUnit Prefix to Multiplier.vi"() -> ("multiplier"=w862:dbl)  [unwired: 1 in, 4 out]
                          n276 = Divide(x=w863, y=w862) -> (x/y=w861:dbl)
                        }
                      }
                      n277 = Bundle("Log Out"=w844, "Log Out"=w841, "z"=w848) -> (w850:cluster{"Log Out":dbl, "Log Out":dbl, "z":dbl})  [unwired: 1 out]
                    }
                    n278 = Unbundle By Name(w827) -> ("display X"=w825:bool, "display Y"=w824:bool, "display Z"=w823:bool)
                    n279 = Bundle By Name(cluster=w835, "single val"=w810, "Name"=w828, "Curve"=w833, "X unit"=w819, "X data"=w814, "X axis"=u16 0 ("X data"), "Y unit"=w818, "Y data"=w815, "Y axis"=w821, "Z unit"=w817, "Z data"=w816, "Z axis"=w821, "X dB ref"=w812, "Y dB ref"=w813, "Z dB ref"=1.0 ("X dB ref"), "display X"=w825, "display Y"=w824, "display Z"=w823) -> (w834:T2)
                    n280 = Build Array (concatenate)(w839, w834) -> (w840:T2[])
                  }
                }
              }
            }
          }
        }
        frame #3 {
          # "0,    Is Standard Error?\n1,    Is Confidence Limits?\n2,    Is Totle Noise?\n3,    Is Har meas.freq?\n4,    Is Total Distortion?\n5,    Is THD?\n6,    Is THD Normalized?\n7,    Is THD Noise?\n8,    Is Rub & Buzz?\n9,  Is Rub & Buzz Norm'd?\n10, Is Perceptual Rub & Buzz? \n11,  Is Total IM?\n12,  Is Total IMD?\n13,  Is Total IMD + N?\n14,  Is Total Diff?\n15,  Is Total DFD(%)?\n16,  Is Total DFD + Noise?"
          n281 = case shown="2, 4" w916 {
            selector: w916 -> [_ w936]
            tunnel: w919 -> [_ w923]
            tunnel: w921 -> [_ w949]
            tunnel: w920 -> [_ w941]
            tunnel: [w922 w945] -> w915
            tunnel: w914 -> [w922 w944]
            tunnel: w913 -> [_ w940]
            tunnel: w918 -> [_ _]
            tunnel: w917 -> [_ w943]
            frame Default {
            }
            frame 2, 4 {
              # "Harmonic and TSR"
              # "????????"
              n282 = Unbundle By Name(w940) -> ("Mic Current"=w924:bool, "use custom unit"=w935:bool, "Imp"=w926:bool, "Type"=w939:u16, "Custom Curve Names"=w934:string[], "Custom Curve IDs"=w933:i32[], "Default Curve Names"=w932:string[], "Use default"=w931:bool)
              n283 = Greater?(x=w936, y=1) -> (0:w946:bool)
              n284 = And(x=w941, y=w946) -> (x .and. y?=w947:bool)
              n285 = local read "HT Option"() -> (w928:bool[])
              n286 = local read "Unit Info"() -> (w942:T6)
              n287 = Build Array(w926, w924) -> (w925:bool[])
              n288 = case shown="2" w936 {
                tunnel: w925 -> [_ w979 w995]
                tunnel: w939 -> [_ w978 _]
                tunnel: [_ w977 w994] -> w930
                tunnel: w943 -> [_ w975 w992]
                tunnel: w942 -> [_ w976 w993]
                tunnel: [_ w974 w991] -> w937
                tunnel: w941 -> [_ w973 w989]
                tunnel: [_ w970 w986] -> w938
                tunnel: w935 -> [_ w968 w984]
                tunnel: w934 -> [_ w967 w983]
                tunnel: w933 -> [_ w966 w982]
                tunnel: w932 -> [_ w965 w981]
                tunnel: w931 -> [_ w964 w980]
                frame Default {
                }
                frame 2 {
                  n289 = local read "HT Option"() -> (w969:bool[])
                  n290 = Bundle(w973, "Check Option"="Independence Order", "use custom unit"=w968, "Custom Curve Names"=w967, "Custom Curve IDs"=w966, "Default Curve Names"=w965, "Use default"=w964) -> (w971:T15)  [unwired: 1 in]
                  n291 = call "CRYGet Harmonics Curve array.vi"("Impedance and Mic Current In"=w979, "Additive Info"=w971, "Option Array In"=w969, "Unit Info"=w976, "Diff array"=w975, "IM array"=w975, "Harmonics array"=w975, "Type"=w978) -> ("Display Array"=w970:T29, "Unit Info Out"=w974:T30[], "Curve Info Array Out"=w977:T31)  [unwired: 1 out]
                }
                frame 4 {
                  n292 = local read "HT Option"() -> (w985:bool[])
                  n293 = Bundle(w989, "Check Option"="Independence Order For TSR", "use custom unit"=w984, "Custom Curve Names"=w983, "Custom Curve IDs"=w982, "Default Curve Names"=w981, "Use default"=w980) -> (w987:T15)  [unwired: 1 in]
                  n294 = call "CRYGet Harmonics Curve array.vi"("Impedance and Mic Current In"=w995, "Additive Info"=w987, "Option Array In"=w985, "Unit Info"=w993, "Harmonics array"=w992, "Type"=u16 0) -> ("Display Array"=w986:T29, "Unit Info Out"=w991:T30[], "Curve Info Array Out"=w994:T31)  [unwired: 2 in, 1 out]
                }
              }
              n295 = for {
                tunnel: w928 -> [w954] mode=indexing
                shift-right: [w953] -> w927
                shift-left: i32[] [] -> [w952]
                i -> [w951]
                n296 = case shown="Default" w951 {
                  tunnel: w954 -> [_ w959]
                  tunnel: w951 -> [_ w958]
                  tunnel: [w955 w957] -> w953
                  tunnel: w952 -> [w955 w956]
                  frame 0..3 {
                  }
                  frame Default {
                    n297 = case shown="True" w959 {
                      tunnel: w958 -> [_ w963]
                      tunnel: [w960 w962] -> w957
                      tunnel: w956 -> [w960 w961]
                      frame False {
                      }
                      frame True {
                        n298 = Insert Into Array(array=w961, new element=w963) -> (w962:i32[])  [unwired: 1 in]
                      }
                    }
                  }
                }
              }
              n299 = call "CRYUnflatten Data.vi"() -> ("Datum"=w950:T2)  [unwired: 1 in, 10 out]
              n300 = for {
                tunnel: w923 -> [w1014] mode=indexing
                tunnel: w950 -> [w1025]
                shift-right: [w1026] -> w945
                shift-left: w944 -> [w1024]
                tunnel: w949 -> [w1023]
                tunnel: w947 -> [w1022]
                tunnel: w938 -> [w1013] mode=indexing
                tunnel: w937 -> [w1009] mode=indexing
                tunnel: w930 -> [w1005] mode=indexing
                tunnel: w927 -> [w1003] mode=indexing
                n301 = Unbundle By Name(w1014) -> ("Harmonic Track Data"=w1021:cluster{cluster{"x":dbl, "y":dbl, "z":dbl}[]}[])
                n302 = Unbundle By Name(w1009) -> ("X dB ref"=w998:dbl, "Y dB ref"=w997:dbl, "Y data Time"=w999:u16, "X data"=w1000:u16, "X unit"=w1008:string, "Y unit"=w1007:string, "Y data Time"=w1006:u16, "single/curve"=w996:bool)
                n303 = Unbundle By Name(w1013) -> ("display X"=w1012:bool, "display Y"=w1011:bool, "display Z"=w1010:bool)
                n304 = Unbundle By Name(w1005) -> ("Custom Curve Name"=w1004:string)
                n305 = local read "Channel Label In"() -> (w1020:string)
                n306 = case shown="True" w1022 {
                  tunnel: w1021 -> [w1063 w1066]
                  tunnel: w1023 -> [_ w1065]
                  tunnel: [w1063 w1064] -> w1015
                  frame False {
                  }
                  frame True {
                    n307 = call "CRYHarmonic curves x-axis replace.vi"("New X axis"=w1065, "Freq resp curves"=w1066) -> ("Freq resp curves out"=w1064:cluster{cluster{"x":dbl, "y":dbl, "z":dbl}[]}[])  [unwired: 9 out]
                  }
                }
                n308 = Index Array(array=w1015, index=0 ("Index")) -> (element=w1017:cluster{cluster{"x":dbl, "y":dbl, "z":dbl}[]})
                n309 = Concatenate Strings(w1004, w1020) -> (w1018:string)
                n310 = Unbundle(w1017) -> (w1002:cluster{"x":dbl, "y":dbl, "z":dbl}[])
                n311 = case shown="4, 10, 13" w1003 {
                  tunnel: w1002 -> [w1027 w1035]
                  tunnel: [w1027 w1034] -> w1001
                  tunnel: w1000 -> [_ w1033]
                  tunnel: w999 -> [_ w1032]
                  tunnel: w998 -> [_ w1031]
                  tunnel: w997 -> [_ w1029]
                  frame Default {
                  }
                  frame 4, 10, 13 {
                    n312 = Multiply(x=1e-50 ("Y dB ref"), y=w1029) -> (x*y=w1028:dbl)
                    n313 = for {
                      tunnel: w1035 -> [w1044] mode=indexing
                      tunnel: w1029 -> [w1046]
                      tunnel: [w1045] -> w1034 mode=indexing
                      tunnel: w1032 -> [w1038]
                      tunnel: w1033 -> [w1042]
                      tunnel: w1031 -> [w1041]
                      tunnel: [w1037] -> _ mode=indexing
                      tunnel: w1028 -> [w1036]
                      n314 = Unbundle(w1044) -> ("x"=w1040:dbl, "y"=w1047:dbl, "z"=w1043:dbl)
                      n315 = case shown="..0" w1038 {
                        tunnel: w1047 -> [w1056 w1062]
                        tunnel: w1046 -> [w1059 _]
                        tunnel: [w1058 w1060] -> w1037
                        tunnel: w1036 -> [w1055 _]
                        frame ..0 {
                          n316 = Less Or Equal To 0?(x=w1056) -> (x <= 0?=w1057:bool)
                          n317 = Select(t=w1055, s=w1057, f=w1056) -> (s? t:f=w1054:dbl)
                          n318 = call "CRYConversion dB-Lin.vi"("dB ref."=w1059, "Lin In"=w1054) -> ("Log Out"=w1058:dbl)  [unwired: 4 in, 3 out]
                        }
                        frame 1.. {
                          n319 = call "CRYUnit Prefix to Multiplier.vi"() -> ("multiplier"=w1061:dbl)  [unwired: 1 in, 4 out]
                          n320 = Divide(x=w1062, y=w1061) -> (x/y=w1060:dbl)
                        }
                      }
                      n321 = case shown="..0" w1042 {
                        tunnel: w1040 -> [w1050 w1053]
                        tunnel: w1041 -> [w1049 _]
                        tunnel: [w1048 w1051] -> w1039
                        frame ..0 {
                          n322 = call "CRYConversion dB-Lin.vi"("dB ref."=w1049, "Lin In"=w1050) -> ("Log Out"=w1048:dbl)  [unwired: 4 in, 3 out]
                        }
                        frame 1.. {
                          n323 = call "CRYUnit Prefix to Multiplier.vi"() -> ("multiplier"=w1052:dbl)  [unwired: 1 in, 4 out]
                          n324 = Divide(x=w1053, y=w1052) -> (x/y=w1051:dbl)
                        }
                      }
                      n325 = Bundle("Log Out"=w1039, "Log Out"=w1037, "z"=w1043) -> (w1045:cluster{"Log Out":dbl, "Log Out":dbl, "z":dbl})  [unwired: 1 out]
                    }
                  }
                }
                n326 = Bundle By Name(cluster=w1025, "Curve"=w1001, "Name"=w1018, "X unit"=w1008, "Y unit"=w1007, "Y data"=w1006, "single val"=w996, "display X"=w1012, "display Y"=w1011, "display Z"=w1010) -> (w1019:T2)
                n327 = Build Array (concatenate)(w1024, w1019) -> (w1026:T2[])
              }
            }
          }
        }
        frame #4 {
          n328 = Unbundle By Name(w1091) -> ("Sampling Rate"=w1090:dbl)
          n329 = Unbundle By Name(w1069) -> ("Signal Type"=w1072:string, "EQ"=w1070:bool, "Level Out2"=w1067:dbl)
          n330 = call "CRYGet Current Calibration Info.vi"("Is Input?"=FALSE, "Signal Type Name"=w1072) -> ("Calibration All Cluster"=w1073:T4)  [unwired: 9 out]
          n331 = Unbundle By Name(w1085) -> ("use custom unit"=w1084:bool, "Custom Curve Names"=w1083:string[], "Custom Curve IDs"=w1082:i32[], "Default Curve Names"=w1081:string[], "Use default"=w1080:bool)
          n332 = Unbundle By Name(w1073) -> ("EQ Curve"=w1071:T2)
          n333 = Bundle("EQ Curve"=w1071, "EQ"=w1070, "Level Out2"=w1067) -> (w1068:T20)  [unwired: 1 in]
          n334 = Unbundle By Name(w1085) -> ("Envelope"=w1125:bool, "impulse"=w1124:bool, "Deconvolved Response"=w1123:bool, "Auto-Correlation(Stimulus)"=w1122:bool, "Auto-Correlation(Response)"=w1121:bool, "Cross-Correlation"=w1120:bool, "Fmin(Hz)"=w1119:dbl, "Fmax(Hz)"=w1118:dbl, "Averaging"=w1110:u16, "Scaling"=w1077:i32, "Freq.Resolution"=w1117:dbl, "Default Overlap"=w1116:bool, "Overlap"=w1115:dbl, "discard cycles"=w1114:dbl, "start ms"=w1113:dbl, "stop ms"=w1112:dbl, "Over-samples Res."=w1111:dbl, "ResponseMe"=w1089:u16, "Loose Particle"=w1098:bool, "Weigting"=w1079:string)
          n335 = local read "Impulse Resp X"() -> (w1105:dbl[])
          n336 = local read "Impulse Resp Y"() -> (w1104:dbl[][])
          n337 = local read "Channel Label In"() -> (w1095:string)
          n338 = local read "TSR window"() -> (w1106:u16)
          n339 = local read "Unit Info"() -> (w1099:T6)
          n340 = local read "Window"() -> (w1107:u16)
          n341 = Bundle("Harmonics array out"=w1102, "Impulse Resp X"=w1105, "Impulse Resp Y"=w1104) -> (w1092:T34)  [unwired: 1 in]
          n342 = Build Array(w1125, w1124, w1123, w1122, w1121, w1120) -> (w1109:bool[])
          n343 = Bundle("Fmin(Hz)"=w1119, "Fmax(Hz)"=w1118, "Averaging"=w1110, "Scaling"=w1077) -> (w1094:T35)  [unwired: 1 in]
          n344 = Bundle("Sampling Rate"=w1090, "Channel Label In"=w1095, "Make Fundamental curve?"=w1100) -> (w1103:T36)  [unwired: 1 in]
          n345 = Bundle("Window"=w1107, "TSR window"=w1106, "Freq.Resolution"=w1117, "Default Overlap"=w1116, "Overlap"=w1115, "discard cycles"=w1114, "start ms"=w1113, "stop ms"=w1112, "Over-samples Res."=w1111, "ResponseMe"=w1089, "Weigting"=w1079) -> (w1108:T37)  [unwired: 1 in]
          n346 = Bundle(w1087, "", "use custom unit"=w1084, "Custom Curve Names"=w1083, "Custom Curve IDs"=w1082, "Default Curve Names"=w1081, "Use default"=w1080) -> (w1088:T38)  [unwired: 1 in]
          n347 = call "CRYAna Time.vi"("Time Option"=w1109, "Graph Info"=w1103, "TSR Info"=w1092, "Additive Info"=w1088, "Stimulus"=w1093, "Input Info"=w1108, "Response"=w1078, "Unit Info"=w1099, "Algorithm"=w1101, "Result Waveform"=w1094, "EQ information"=w1068) -> ("Wave out"=w1096:T7[])  [unwired: 4 in]
          n348 = case shown="True" w1098 {
            tunnel: w1099 -> [_ w1145]
            tunnel: w1097 -> [w1126 w1144]
            tunnel: [w1126 w1128] -> w1076
            tunnel: w1096 -> [w1127 w1142]
            tunnel: [w1127 w1140] -> w1075
            tunnel: w1095 -> [_ w1139]
            tunnel: w1085 -> [_ w1138]
            tunnel: w1078 -> [_ w1131]
            tunnel: w1090 -> [_ w1130]
            frame False {
            }
            frame True {
              n349 = Unbundle By Name(w1138) -> ("Attack Threshold"=w1133:dbl, "Averaging Time"=w1137:dbl, "Max duration"=w1136:dbl, "Min duration"=w1135:dbl, "Hysteresis Up"=w1134:dbl)
              n350 = Bundle("Attack Threshold"=w1133, "Averaging Time"=w1137, "Max duration"=w1136, "Min duration"=w1135, "Hysteresis Up"=w1134, "Loose Particle"=TRUE) -> (w1132:T39)  [unwired: 1 in]
              n351 = call "CRYAna Loose Particles.vi"("Loose part"=w1132, "Unit Info"=w1145, "Fs"=w1130, "Response"=w1131, "Channel Label In"=w1139) -> ("Value Out"=w1143:T2[], "Wave out"=w1141:T7[])  [unwired: 5 in]
              n352 = Build Array (concatenate)(w1142, w1141) -> (w1140:T7[])
              n353 = Build Array (concatenate)(w1143, w1144) -> (w1128:T2[])
            }
          }
        }
      }
      n354 = Build Array (concatenate)(w105, w117) -> (w50:T2[])
      n355 = for {
        tunnel: w50 -> [w161] mode=indexing
        tunnel: w101 -> [w167]
        shift-right: [w162] -> w92
        shift-left: w48 -> [w165]
        shift-right: [w164] -> w93
        shift-left: w48 -> [w163]
        tunnel: [w159] -> w38 mode=indexing
        n356 = Unbundle By Name(w161) -> ("single val"=w166:bool)
        n357 = Bundle By Name(cluster=w161, "Step No."=w167, "Test Info"="") -> (w159:T2)
        n358 = case shown="True" w166 {
          tunnel: w159 -> [w169 w172]
          tunnel: w165 -> [w171 w174]
          tunnel: [w168 w175] -> w164
          tunnel: w163 -> [w170 w175]
          tunnel: [w171 w173] -> w162
          frame False {
            n359 = Build Array (concatenate)(w170, w169) -> (w168:T8)
          }
          frame True {
            n360 = Build Array (concatenate)(w174, w172) -> (w173:T8)
          }
        }
      }
      "Data out" <- w38
      n361 = for {
        tunnel: w115 -> [w158] mode=indexing
        tunnel: w101 -> [w157]
        tunnel: [w156] -> w83 mode=indexing
        n362 = Bundle By Name(cluster=w158, "Step No."=w157) -> (w156:T7)
      }
      "Wave out" <- w83
      n363 = Bundle By Name(cluster="Result", "Verdict"=TRUE, "Step No."=w101, "Name"=w45) -> (w110:T1)
      n364 = global read "CRYProject Run Control Global.vi" "RunState"() -> (w89:bool)
      n365 = Build Array(w110) -> (→"Results out":T1[])
      n366 = case shown="True" w89 {
        tunnel: ["Apply" ("sOption1") "Run" ("Type In")] -> w87
        tunnel: ["APPLY_CURVE" ("Type In") "RUN_CURVE" ("Type In")] -> w88
        frame False {
        }
        frame True {
        }
      }
      n367 = Index Array(array=w97, index=1) -> (element=w91:bool)
      n368 = Index Array(array=w38, index=1) -> (element=w37:T2)
      n369 = Select(t="Overwrite" ("Y unit"), s=w91, f="Repeat") -> (s? t:f=w96:string)
      n370 = case shown="False" w91 {
        tunnel: w93 -> [w147 w150]
        tunnel: w92 -> [w146 w149]
        tunnel: w83 -> [w145 w148]
        tunnel: [w144 w150] -> w42
        tunnel: [w143 w149] -> w41
        tunnel: [w142 w148] -> w40
        tunnel: w90 -> [w141 _]
        tunnel: w88 -> [w140 _]
        frame False {
          n371 = call "CRYPrefix Curve Name.vi"("Type In"=w140, "Curves In"=w147, "Values In"=w146, "Waves In"=w145, "Repeat State Array In"=w141) -> ("Curves Out"=w144:T8, "Values Out"=w143:T8, "Waves Out"=w142:T40)  [unwired: 7 in, 1 out]
        }
        frame True {
        }
      }
      n372 = Unbundle By Name(w37) -> ("Curve"=w35:cluster{"x":dbl, "y":dbl, "z":dbl}[])
      n373 = for {
        tunnel: w35 -> [w122] mode=indexing
        tunnel: [w121] -> w34 mode=indexing
        tunnel: [w120] -> w33 mode=indexing
        n374 = Unbundle By Name(w122) -> ("x"=w121:dbl, "y"=w120:dbl)
      }
      n375 = call "CRYInsert Socket.vi"("sOption2"=w96, "Step No."=w101, "sOption1"=w87, "Waves"=w40, "Values"=w41, "Curves"=w42) -> ("Inserted Names Out"=→"Inserted Names Out":string[])  [unwired: 5 in]
      n376 = call "CRYGet Type from Data.vi"("Waves"=w40, "Values"=w41, "Curves"=w42) -> ("Type"=→"Types Out":string[])  [unwired: 8 in]
      n377 = Bundle(w34, w33) -> (→"XY Graph":cluster{dbl[], dbl[]})  [unwired: 1 in]
    }
  }
